vi "pylon_FSRS1.vi"() -> ()   [LabVIEW 2014]
uses:
  Public/Documents/SIToolkit/LabVIEW/Examples2014_6_0_2_9/Fast Examples/Open-Close Hardware/CamHandle.vi
  <vilib>/Utility/file.llb/Write To Spreadsheet File (I64).vi
  <vilib>/Utility/file.llb/Write To Spreadsheet File (DBL).vi
panel:
  in  "?":enum32{"CONFIGURATION", "OPERATION"}(tab)=enum."OPERATION"
  in  "Bypass Cooling":bool
  in  "Write Tab Control":T1(tab)=enum."ROI"
  in  "Frames to collect (nframe)":u32=1 min=1 step=1
  in  "Exposure":dbl min=0.0 step=0.001 format="%.3f"
  in  "Timing Mode":u32(ring)=3 items=["Free Run/Timed"=1, "External Sync"=3, "Shift per Trigger"=13]
  in  "Trigger Edge":u32(ring)=1 items=["Positive Edge"=1, "Negative Edge"=2]
  in  "Collection Mode":u32(ring)=1 items=["Focus"=1, "N-Frame"=2, "Asynchronous"=3]
  in  "Readut Mode":u16(ring)=1 items=["Full Frame"=1, "Kinetics"=10]
  in  "Temperature":dbl=-75.0 format="%.2f"
  in  "Speed":i32=-2 min=-3 step=1
  in  "Gain":i32(ring)=3 items=["Don't Change "=-1, "Low"=1, "Medium"=2, "High"=3]
  in  "Offset":i32=-1 min=-1 step=1
  in  "Readout Port":i32(ring)=2 items=["Don't Change"=-1, "Low Noise"=1, "High capacity"=2]
  in  "Open":u32
  in  "Close":u32
  in  "Shutter State":u16(ring)=3 items=["Always Closed"=1, "Open Each Exposure"=2, "Open at Begining of Acquisition"=3, "Open While Waiting for Trigger"=4]
  in  "Minium Block Size":u32=1
  in  "Number of Minimum Blocks":u32=1
  in  "Number of Clean/Clears cycles":u32
  in  "Number of Strips per Clean":u32=100
  in  "Continous Cleans":bool
  in  "Skip Serial Register Clean":bool=TRUE
  in  "Kinetics Window Height":u32
  in  "Active Y Size":u32=100
  in  "Post Y":u32=8
  in  "Pre Y":u32=8
  in  "Active X Size":u32=1340
  in  "Post X":u32
  in  "Pre X":u32
  in  "Vertical Timing Index":u32
  in  "Enable  Custom Chip":bool=TRUE
  in  "Logic Output":u16(ring)=3 items=["Not Scan / Not Reading"=1, "Shutter Open"=2, "Not Ready/Busy"=3, "Always Low"=4, "Always High"=8]
  in  "Invert":bool
  out "Y Size ROI":u32=100
  out "X Size ROI":u32=1340
  in  "Y Bin":u32=100 min=1 step=1
  in  "Y End":u32=100 min=1 step=1
  in  "Y Start":u32=1 min=1 step=1
  in  "X Bin":u32=1 min=1 step=1
  in  "X End":u32=1340 min=1 max=100000 step=1
  in  "X Start":u32=1 min=1 step=1
  in  "Error Codes":string="Ready"
  out "Frame Rate":dbl=1001.0010010010011
  out "Vertical Index":u32
  out "Custom Chip Enabled":bool
  out "Vertical Timing":dbl=3.2
  out "Readout Time":dbl=0.9989999999999999
  out "Temperature":dbl=-75.0
  out "Pixel Time":i32=500
  out "Bit Depth":i32=16
  out "ReadOut Port":i32=2
  out "ADC Offset":i32=-1
  out "ADC Gain":i32=3
  out "ADC Speed":i32=2000
  in  "error in (no error)":errorcluster
  out "error out":errorcluster
  out "Camera Handle":u32=16842752
  in  "INI Flag":bool=TRUE
  in  "Camera Number":u32=1
  in  "?":enum32{"RUN", "FOCUS", "FSRS", "SPECTROGRAPH"}(tab)=enum."FOCUS"
  in  "?":bool
  in  "Exposure Time (s)":dbl=0.004 min=0.0 step=0.001 format="%.3f"
  in  "?":bool
  in  "?":bool
  out "?":u16[](graph)
  in  "file path":path
  in  "File_name":string
  in  "# of spectrum per frame":i32
  in  "# of Frames":i32
  out "Gain":dbl=14.743310504423635
  in  "FLIP SPECTRA":bool
  in  "?":bool
  in  "?":bool
  in  "?":bool
  out "Spectra":dbl[](graph)=[0.9755300872844695, 0.9756768462539598, 0.97581696418543, 0.9762743991329165, 0.9751930768187929, 0.9752114673732061, 0.9751177936489209, 0.9764930270973735, 0.9763887386039467, 0.9749810931230943, 0.9742926745030784, 0.9759744997206772, 0.9754796564203729, 0.9761178908183206, 0.9752425241815373, 0.9766219750252831, 0.9761877743519881, 0.9761361753868542, 0.9776978491334654, 0.9779277019501946, 0.977147036323896, 0.9792513539762008, 0.9795268534910172, 0.9787884146751874, 0.9804470957694494, 0.982035881204582, 0.982528667778694, 0.9825823402901814, 0.9843882822979847, 0.9839266633595681, 0.9849468846920538, 0.9872698212511262, 0.988122544550336, 0.9877812802972845, 0.9885869980663688, 0.9900703844600179, 0.9927077538710171, 0.9932628998596844, 0.9932460798479855, 0.9935570775182174, 0.9945507204569972, 0.9951647818460134, 0.9962848374908384, 0.9972893370585736, 0.9965515155280157, 0.9984594060832435, 0.9973443014380436, 0.9989028091476645, 0.9990774165831509, 0.9983506095949803, 1.0007898394202042, 0.9991913406017616, 0.9992492731339196, 1.0010480478392645, 0.999582213532268, 0.9991496850542972, 1.0003341169724274, 1.0007777101312207, 0.9999823435413888, 1.000981058256019, 1.00207813229889, 1.0016715850846636, 1.0016509685396446, 1.0023107232087645, 1.0018617734738753, 1.002175650976147, 1.0016212316773503, 1.002062777617173, 1.002372669657128, 1.0023120696051897, 1.0022985765507009, 1.0023149704491137, 1.0021015205484045, 1.0017074421552823, 1.0023106670699446, 1.0032785517995444, 1.0018856636029874, 1.0032932634895588, 1.0028768911229609, 1.003726073257663, 1.0036399397267421, 1.0033806164078303, 1.0041437793153363, 1.0037179628801496, 1.0033493482112539, 1.0037501476114246, 1.0042959964606617, 1.0042755419219582, 1.0048754785866216, 1.0047939316440613, 1.0053694568681872, 1.0038757728966237, 1.0048674931155683, 1.0047690942831697, 1.0051252430535689, 1.0053741704915389, 1.0049524139095343, 1.0045025426639995, 1.0040228927138426, 1.0039933320314238, 1.0041510866852374, 1.0033303068586903, 1.003533250646326, 1.0027459506237124, 1.0026057826647117, 1.003260830428883, 1.0032007978706163, 1.0026495289070276, 1.0021436528670513, 1.0028330294934311, 1.00231600280275, 1.0012086967393559, 1.001014014161519, 1.0015504074851016, 1.0009696535006722, 1.0019791149958475, 1.0011346392927039, 1.0012359758891582, 0.9998570077525675, 1.0010428549273014, 1.0009149466593552, 1.0002830176584063, 0.9994048138652198, 1.0002597870365144, 1.0003278859881963, 0.9995526733478612, 0.999438177342597, 0.9998261877083351, 1.0010865765016752, 1.0000489926845766, 1.0008545626290852, 1.0008522612809412, 1.0010707079783248, 1.001090857433441, 1.0008982925251158, 1.003486669845695, 1.0047949174912858, 1.0077445761417212, 1.0120141741517803, 1.0201772595698257, 1.0322536760974164, 1.0501541199055933, 1.0754172950855931, 1.1067885797289987, 1.1374285660931862, 1.1481866653218364, 1.1326606889231363, 1.09741400039275, 1.0612674001718378, 1.0350214908693538, 1.0206930861271215, 1.0139256277018351, 1.0089963920346658, 1.0060688393052548, 1.0052123238345017, 1.0028067604394633, 1.0012638696493386, 1.0013393221695588, 0.9985981192113675, 0.9987380376267128, 0.9979073384358298, 0.9967424944898179, 0.9966884820000458, 0.9963776196534506, 0.9960720866862709, 0.9965830445533452, 0.9977931108410204, 0.9985995492168933, 0.9986199775849548, 0.9987633729071931, 0.9984312093430782, 0.9997148642087165, 0.9996065463963878, 0.9998582689274716, 1.0002110852616093, 1.0000077618826129, 1.0000489132335226, 1.0003573806378223, 0.9999187010432274, 1.001963517608326, 1.0012593397700642, 1.0018807550628366, 1.0031660227654289, 1.0020918035773498, 1.0028275747471433, 1.0028088790557186, 1.0025566510225332, 1.0023556237093005, 1.0032096086622704, 1.0017564747987622, 1.0035091544995398, 1.0017366497034703, 1.0019443199711786, 1.0020298982939733, 1.0013981641538263, 1.0010735915908218, 1.001793476880256, 1.0022368226440215, 1.0014151948414793, 1.0017759582228316, 1.0014962508125689, 1.0018072606384634, 1.0000417440167613, 1.0005621657797237, 0.9998446426790336, 0.9998454860152206, 1.0001492253861217, 0.9994421154150686, 0.9995411675602213, 0.9987441278717668, 0.9998158390779703, 0.9988418583687989, 0.9993341276421205, 0.9990993990819101, 0.9990807904190898, 0.9983948439832072, 0.9985400716676921, 0.9985927240493662, 0.9982560336788509, 0.9982625964427206, 0.9985155142344474, 0.998404835032493, 0.9979263060413635, 0.9982868928614334, 0.9973870564732009, 0.9978861496786271, 0.9978082037249373, 0.9976350693353202, 0.9978557947960519, 0.9992941525783824, 0.9975784845094273, 0.9980438675332602, 0.9973132560896502, 0.9983960703496668, 0.9975817679789122, 0.9970631933860724, 0.9968645888999441, 0.9969550208616594, 0.9968574087836076, 0.9962806908544759, 0.996370069484568, 0.9981588855574023, 0.9971286326512906, 0.9968130048156779, 0.9967659060092784, 0.9962581267842879, 0.9973137060022212, 0.9964871894740839, 0.9965162310427663, 0.996997193641602, 0.9965704833779099, 0.9963915930394757, 0.9962108827034403, 0.9960472238857022, 0.995857865398809, 0.9961579582249456, 0.9971978885120082, 0.9961331760017116, 0.996721337440865, 0.9965996253465066, 0.9965304002168622, 0.9956403635637245, 0.9955790038812106, 0.9956912830823886, 0.9949089431758003, 0.9946282645549207, 0.9934605416581226, 0.9927704057498754, 0.9935944194028669, 0.991876783433561, 0.9926946308356118, 0.9932993795948648, 0.9943894372954812, 0.9936112074994828, 0.9939246568355098, 0.9935242137901221, 0.9936503123346356, 0.9936963818576866, 0.994682882264595, 0.9937856190284484, 0.9940832926061379, 0.993164306278515, 0.9940404284685382, 0.9937880441864195, 0.9942411288661716, 0.9928753466028547, 0.9950984658310266, 0.9927277176741094, 0.9940334005450226, 0.9929660360364769, 0.9930487414589113, 0.9935365540438033, 0.9934139033392642, 0.9928950534503354, 0.9929034314029997, 0.9937174013031602, 0.9923612045121255, 0.9925908921890753, 0.9932679282052643, 0.9935763003400074, 0.9931199695791296, 0.9929887699255886, 0.9918197209507501, 0.9917853379343897, 0.9921991173870989, 0.9935339294252353, 0.9925704988068781, 0.9917055357360344, 0.992014507869348, 0.9917718012401779, 0.9909311230807839, 0.9909039735016065, 0.9896572589564085, 0.9891350823517422, 0.9894682209515745, 0.9888525713434655, 0.9909080023425957, 0.9912954671309397, 0.9935124803850233, 0.9938587756634525, 0.9946849857860757, 0.996592195888077, 0.9968503534981081, 0.9973935731820813, 0.9989584060578116, 1.0019087222262957, 1.0049043836984641, 1.0080586432045664, 1.009751294323102, 1.012303874345489, 1.0129703221236666, 1.013272938321382, 1.011503753925153, 1.0105758873330835, 1.0075438150818337, 1.0057435426202306, 1.0041342342197446, 1.0026209652997937, 1.0005848295336346, 0.9994019123146808, 0.9991868572532903, 0.9977512308696675, 0.9970075134065679, 0.9966356360857342, 0.9959060548781977, 0.9964393102123654, 0.9958649592771627, 0.9950662281056751, 0.9953116557885184, 0.9948664403448791, 0.9947278335757348, 0.9939669263212532, 0.993667523914121, 0.9945029544068963, 0.9936192521599826, 0.9921074321024335, 0.9914254678032394, 0.9903272540137805, 0.9892925938271362, 0.9887848718524774, 0.9893134788695674, 0.9882838661440005, 0.9895055869783085, 0.9891480148597968, 0.9884337022120356, 0.991156915494973, 0.9896733386520254, 0.9893394415489665, 0.9904097944203936, 0.9902381774153993, 0.9901524278073909, 0.9900581421557813, 0.9905585242206175, 0.9908406929910862, 0.9915079648120938, 0.9906566524112734, 0.9911394696363427, 0.9916113980702473, 0.9910989259973373, 0.9903792532358182, 0.9907827317977844, 0.9905977304469169, 0.991456239330327, 0.9916819598107186, 0.9914199515036257, 0.9906942610155813, 0.9926315563028391, 0.9914270997426113, 0.9915539601421401, 0.9912235268405463, 0.992088607849578, 0.9913444613666713, 0.991908492679886, 0.9915866831630165, 0.9919952301201026, 0.9932504567792872, 0.9921046559674063, 0.9924291983048888, 0.9916447610149356, 0.991848590750747, 0.9921425513517983, 0.9919714570173391, 0.9925466399620982, 0.9928838907426037, 0.9924196088955134, 0.9931616675611925, 0.9927461163593102, 0.9931309100549827, 0.9934496416081131, 0.9927927896501221, 0.9934964738267893, 0.9928551133908948, 0.9942999569046416, 0.9931792408327563, 0.9925693415358496, 0.9934360330716882, 0.9949747557474269, 0.993731157710846, 0.9938433747596407, 0.994740733427746, 0.9943609592519476, 0.9943541746199618, 0.9939486211816836, 0.992950149807933, 0.9941678883691097, 0.9943180628327398, 0.99513015651641, 0.9943919298791273, 0.9941424826530518, 0.9936525300481539, 0.9949917538640838, 0.9955375244736728, 0.9951439299329877, 0.9962050263298082, 0.9963947799134774, 0.9968244979975278, 0.9983975806265784, 1.000533927758882, 1.0029408707991847, 1.0048711521008775, 1.0068304778141166, 1.007018989034806, 1.0029759503979807, 1.0000482254275387, 0.9975549973629185, 0.9974036736573202, 0.9968789927911186, 0.9960748811206702, 0.9965189333035787, 0.995140250519678, 0.9958415984118337, 0.9949389664472165, 0.9949181303181669, 0.9952042060002814, 0.9945451790485715, 0.9952437023373856, 0.994276227548833, 0.9953156888749304, 0.9942260097126655, 0.9957965248601841, 0.9946261743510755, 0.9954561818541723, 0.9950439277931782, 0.9947499204338731, 0.9946841217392777, 0.9950829252266876, 0.9954281866903525, 0.9944531747199533, 0.9950511330771304, 0.9948849293283386, 0.9952587470138156, 0.9942422382648602, 0.9926478162749266, 0.9941745367956879, 0.9937302385520251, 0.9943405037447987, 0.9940163977879987, 0.9935998700562014, 0.9939924261400744, 0.9938600227368913, 0.9942658538803476, 0.9941555176670761, 0.9943854145798364, 0.9937595474775596, 0.9942601839347238, 0.9941192503118871, 0.9939902692064626, 0.9939594250617401, 0.9938728119504552, 0.993650669917967, 0.9946982680767041, 0.9943281028619699, 0.9939645957455999, 0.9935648856308205, 0.9941752901094008, 0.9937357059814677, 0.9933247297715599, 0.9938906929289909, 0.9941043870750722, 0.9947695896697957, 0.9926702752126659, 0.9925736732160917, 0.99412276123165, 0.993005018245409, 0.9928841805326482, 0.9928156349036281, 0.9925723613309926, 0.9918506118756122, 0.9911125441857309, 0.9907333399491967, 0.9921429405981673, 0.9905810846498307, 0.9918787814012708, 0.9920241514653586, 0.9918653459895168, 0.9915914658868445, 0.992110337597804, 0.9923605206196495, 0.992686464882264, 0.9938726051269021, 0.9934677141593928, 0.9947213941988519, 0.9939523884200137, 0.9958435480641371, 0.9960878435035664, 0.998112647651406, 0.9976058258921943, 0.9992725956143081, 1.0005451377173482, 1.002641821904002, 1.0041158281009654, 1.0073714634187072, 1.0096194442337205, 1.011401650626004, 1.013070646872337, 1.0119185527223444, 1.0099088327766466, 1.009814022494501, 1.0063825249878426, 1.0032604349198055, 1.0027766338798774, 1.000287952720255, 0.9986277641920462, 0.9980477820943987, 0.9960662676711914, 0.9967893361260675, 0.9952254802975962, 0.9939518521938141, 0.9925135524883861, 0.9926959373886529, 0.9908518984681769, 0.9911725762303055, 0.9906085031171179, 0.9904494224857862, 0.9884528287629935, 0.9887177600890857, 0.9886703754231349, 0.9881853417399994, 0.9881302842296761, 0.9880208726978792, 0.9872135553097768, 0.9871836120110088, 0.9871291081351026, 0.9865338537476699, 0.9859219777639733, 0.9869134352439242, 0.9862738473151121, 0.985608104834756, 0.9867729622891286, 0.9859698167157214, 0.984919024605055, 0.9861937432678872, 0.9848322799791898, 0.9852044388456488, 0.9853417405353183, 0.9835531029615663, 0.9844598200282393, 0.9845169921245397, 0.9843776090258691, 0.9838987127482762, 0.9826194218261648, 0.9834471979752251, 0.9829395469239401, 0.9841809517721625, 0.982740266779254, 0.9832266794850923, 0.983597461693007, 0.9839050454399203, 0.9831586562985791, 0.9832238806837683, 0.9819891319177596, 0.9830146076513276, 0.9823739806909814, 0.9834248081882394, 0.982774720138555, 0.982731503435003, 0.9825121425219699, 0.9833991472534351, 0.982186136274627, 0.9826987591820081, 0.9829784313378913, 0.9840304061865316, 0.984920420832576, 0.9848016580142605, 0.984637173220356, 0.9841012255373592, 0.9845778413710072, 0.9844496403226004, 0.9849069993604949, 0.9840818986135075, 0.9838231864024809, 0.9841145257461423, 0.9834942502404114, 0.9833176167594164, 0.9825157102760381, 0.9819735573764853, 0.9829622528276347, 0.9824945822519466, 0.9800824624551667, 0.982870582958771, 0.9825981856262659, 0.9811956732852909, 0.9822624974687129, 0.9812600672546186, 0.9811591777781735, 0.9819534555557126, 0.9806681085499535, 0.9820342971216329, 0.9813579712911087, 0.9820105505538734, 0.9812343611503167, 0.9816313053027922, 0.9820953937828902, 0.9818152492770197, 0.982330765326644, 0.9814479080657366, 0.982110291220737, 0.9806881232552964, 0.9813703402444995, 0.9821895930373158, 0.9825646178286225, 0.981722882417567, 0.9808083213760249, 0.9816826966365202, 0.9831621913409136, 0.9834519852435336, 0.9819530727831046, 0.9823086743012107, 0.9811220426873025, 0.9812482776238972, 0.9827616800346425, 0.9816851891281408, 0.9813153523769537, 0.9834752237380378, 0.9827038521339388, 0.9831869462124827, 0.9837131268255906, 0.9835637613733392, 0.9825685959375935, 0.9835166246680233, 0.9832899459313126, 0.9821619515717059, 0.9848076338921278, 0.9847424893389772, 0.9841309907479139, 0.9847567871515419, 0.9850805177341108, 0.9840332666925127, 0.9856517840958284, 0.9852222998421788, 0.9856666370667512, 0.9864656814948044, 0.9864209936998543, 0.9878172455904856, 0.9880923255936395, 0.9879512362506478, 0.9885068151698244, 0.989128852007672, 0.9887875769589333, 0.9903708567833138, 0.9900511597787641, 0.9898866071468287, 0.9910275374663167, 0.9914860580416507, 0.9925235006961411, 0.9934471447697623, 0.992608252890163, 0.9951783603126805, 0.9980690075623835, 0.9997639333483898, 1.0010665261241487, 1.002430117428686, 1.0020378147127487, 1.0024980899377627, 1.003737773795738, 1.003249051965976, 1.0002194898909202, 0.9990676595023753, 0.9997259706911115, 0.9969388880023595, 0.9957886841507878, 0.9949867408433444, 0.9953954712618904, 0.9936892062542492, 0.993787433290812, 0.9927546672218368, 0.9928893848791186, 0.9925505392102796, 0.9919471661238599, 0.9934570741748587, 0.9937581848770279, 0.9938985920841611, 0.9923185810211319, 0.9943203693140323, 0.9927044973731295, 0.9925078841695358, 0.991285249799347, 0.9925814458117747, 0.9920082293903025, 0.9921409103620292, 0.9935239939757422, 0.992042032121975, 0.991648559703939, 0.9908100594812931, 0.991996668188471, 0.992115081667455, 0.9935499502402744, 0.9921610012413922, 0.992613755742525, 0.9926860544649216, 0.9931843498730183, 0.992118950616697, 0.9931345665088376, 0.9929109347534303, 0.9930572874896546, 0.9932882948815863, 0.993410070354816, 0.9928699423061463, 0.9928931278711759, 0.9924935984745651, 0.9919420343529557, 0.9949051239072446, 0.9923959438550337, 0.9931297846797755, 0.9934610282296891, 0.9922733950845375, 0.9933423129100107, 0.993633885814162, 0.9953413726408745, 0.9956784502362345, 0.9933450393933152, 0.9939926632528363, 0.9943011106654097, 0.9936895637345653, 0.9941530739146468, 0.9936349646658799, 0.9951285340555722, 0.9950972434060573, 0.992825270720686, 0.993383955751042, 0.9945219100961133, 0.9958067541327413, 0.9956233330801973, 0.994599795734717, 0.9957142187668172, 0.9952556472687264, 0.9953656877312194, 0.9946059001794542, 0.9945539643403842, 0.9962165018925121, 0.9954940183694436, 0.9946000295948717, 0.9964193418537554, 0.9949433708136919, 0.9945754853372089, 0.9948482283130354, 0.9969224697155514, 0.9958301102585727, 0.9960699859491319, 0.994981300144576, 0.9945786563610373, 0.9951551229643493, 0.9967508501720332, 0.9963034128905163, 0.9947019215592646, 0.9965787553169893, 0.9947681378143812, 0.9981260029600254, 0.9966090075869397, 0.9966873532798938, 0.9978610764780583, 0.9969297851191489, 0.9971178057933737, 0.9976647956140443, 0.9969046818611058, 0.9971255060352899, 0.9975130234326345, 0.9960516439088403, 0.99603733180533, 0.9974251622558911, 0.9978872483995073, 0.9970739386760539, 0.99930097772978, 0.995973135092528, 0.9989070331896059, 0.9979431944896187, 0.9962574318221076, 0.998284874712051, 0.9980507065885973, 0.9985778477115815, 0.9968881257036589, 0.9979917702197649, 0.9973169278119626, 0.9974323242885285, 0.9990460618991827, 0.9967916827968758, 0.9981135977737259, 0.9978829186523762, 0.9984133201845818, 0.9973040804544807, 0.9961838114111818, 0.9975563640395146, 0.996994322790135, 0.9941276195898406, 0.9983641002927954, 0.9973307539794544, 0.9974205389337224, 0.9973560126820389, 0.9974096738250385, 0.9988189450338115, 0.9961266693760946, 0.9953281298493775, 0.9974017870532675, 0.9973856781928138, 0.9976341196873302, 0.9967046783619647, 0.9969271039427557, 0.9966967454536432, 0.9979490763684615, 0.9953698577234567, 0.9975806387238231, 0.9977016134759747, 0.9985985697493704, 0.9972305476775422, 0.9967101952847037, 0.9971668005388673, 0.9964289730529284, 0.9955644243748356, 0.9959966886630661, 0.995644758687583, 0.9961616433874917, 0.9967792446201315, 0.9955099897474771, 0.9958855279549809, 0.9954476218405081, 0.9965164632663351, 0.9950987472418618, 0.9955500463495174, 0.9960084036614891, 0.9967133506266788, 0.9949838569402805, 0.9953870910750532, 0.9957161964914851, 0.9955189418471003, 0.9952780736915173, 0.9943982047829744, 0.9958594554531327, 0.9951692159641307, 0.9972328017427001, 0.9950296264899483, 0.9953994162394338, 0.9943475666868853, 0.9952644359541133, 0.995447987953035, 0.9942957701523145, 0.994689648871326, 0.9945194145312566, 0.994398451524699, 0.9933776478611506, 0.9949624280070588, 0.9942830700740656, 0.9931776278224557, 0.9923574560898841, 0.9930554951075137, 0.9946804934635376, 0.9955965668939963, 0.9954263404790484, 0.9936251677674021, 0.9925990628645381, 0.9927432773738994, 0.9935199751181003, 0.9925849730240551, 0.9930033516252744, 0.9928205912875862, 0.9909096801217612, 0.9927703039575004, 0.9911207290263226, 0.9936811659787461, 0.9922899870293168, 0.9914100350152775, 0.9921318011951723, 0.9923914376100682, 0.9917196412768485, 0.9911298413282991, 0.9921835901118113, 0.991389162165264, 0.9900308337285773, 0.9907843437132138, 0.9907360707276159, 0.9915303321538369, 0.9910914841449963, 0.9916721085335287, 0.9905147575837829, 0.9885475299200459, 0.9889453642989275, 0.9905817815731635, 0.9902133936178602, 0.988242707738733, 0.9888230852293703, 0.9888416376753377, 0.9897403338911375, 0.9889867106471915, 0.9908277720228965, 0.9897520943960653, 0.9885535791196446, 0.9893233849009734, 0.987815837986452, 0.9878231875051255, 0.9892981374801907, 0.9873831102432441, 0.9883688597489069, 0.9870737497954729, 0.9882750727641025, 0.9892368384624726, 0.9885509311823762, 0.9877328596549173, 0.988031467066814, 0.9886629145954128, 0.9869863870033517, 0.9891492312967063, 0.9862047702357074, 0.9846632856681823, 0.9857502292131517, 0.9853621145521789, 0.9875959785273185, 0.9865328093925239, 0.9868745911941753, 0.9881208793203661, 0.9875637100247531, 0.987473573375884, 0.9846613464121071, 0.9862682448151167, 0.9859936099978158, 0.9877745806584477, 0.9872523351842334, 0.9884633919606788, 0.9878702817787882, 0.9871517835946108, 0.9873182717255755, 0.9869426138212118, 0.9870630928749186, 0.9868782191180008, 0.9866290342010844, 0.9871063632126472, 0.9870767387478339, 0.9892100304806183, 0.9856950020152947, 0.9862725203091884, 0.988963026427355, 0.98713237033965, 0.9871161785494531, 0.9887067533194143, 0.9851151639884772, 0.9872035949066793, 0.986074022015706, 0.9898358190650977, 0.9893426317428032, 0.9865967008566036, 0.9869508361679556, 0.9856394191868602, 0.9884856255992025, 0.9894815163256031, 0.9882529855875178, 0.9868192366411398, 0.9861315958941457, 0.9893630527665666, 0.9868384497720943, 0.9861536189984526, 0.9888178566241863, 0.9867579453720804, 0.987179733246874, 0.9881337364604343, 0.988627432271096, 0.9893363760375293, 0.9884977254771453, 0.9866357360169483, 0.9890432499899394, 0.9853708868622296, 0.9882718264694069, 0.9856002495340267, 0.9883093383137328, 0.9893738708532213, 0.9892222089472598, 0.9896322650924652, 0.9890899936356693, 0.9859116003714216, 0.9876200119407457, 0.9880123989427891, 0.9890238550127071, 0.9877997133543077, 0.9858156669365054, 0.988452075032815, 0.9874384552105305, 0.9852668216716264, 0.990420592763384, 0.986812319833311, 0.9872746702372613, 0.9884135283243309, 0.9898559858934276, 0.9853195046285885, 0.9882116666588994, 0.988836326416156, 0.9889951277543007, 0.9889739755936575, 0.9892999397960774, 0.9890183107271877, 0.9886904943679752, 0.9893025055256274, 0.9883530237311077, 0.9904523864862361, 0.9895924113847931, 0.9882124261702746, 0.9886951765024136, 0.9872263635916005, 0.9911316500287568, 0.9903100332934901, 0.9900921332468797, 0.9908740072799542, 0.9878369893796128, 0.9904378517826975, 0.9941283419233133, 0.9904646678151535, 0.9904861383307207, 0.9899567607865835, 0.9894396209657828, 0.9891584605747445, 0.9912651432019383, 0.9881619592777285, 0.991769579354686, 0.9897143909164129, 0.9892295794789044, 0.9919979753672009, 0.9900968712395756, 0.9903607410161109, 0.990591273311813, 0.98915183511616, 0.9909957276467207, 0.9893142228087654, 0.9914818720029506, 0.9909371177919686, 0.9899079877928816, 0.9895822415817643, 0.9902121865405016, 0.9895690295265566, 0.9875805843320437, 0.9896141479065251, 0.9904862852268639, 0.9914162763875078, 0.991266180924169, 0.9900029401520938, 0.9919999062371018, 0.9924424015884847, 0.9908311716147565, 0.9922420543168002, 0.990948525584296, 0.991385538920927, 0.9897883622343855, 0.9919614812445081, 0.9902281707455857, 0.994894236690351, 0.9909491027501054, 0.9922156201249668, 0.9902288111203057, 0.9905311413181366, 0.9938940171329753, 0.9901016036840101, 0.9915677278694006, 0.9913941890768317, 0.9909395295168169, 0.9955689263522823, 0.9922709650971144, 0.9922278347497557, 0.9909074461652106, 0.9933836875407083, 0.9939377700843446, 0.9938960186208253, 0.9915969179004076, 0.9936655476411831, 0.9919779969563804, 0.9929206399541289, 0.9921486094292173, 0.9926496485478737, 0.9912891600854369, 0.992964299640567, 0.992144221783553, 0.9939411134849978, 0.9907431243871444, 0.9936131765393752, 0.9936041064577842, 0.9937652534212517, 0.9903211389560228, 0.9917327216280427, 0.9921648683304255, 0.9951627294683641, 0.9922283830374052, 0.9943289558409931, 0.9907424411869826, 0.9955227545424469, 0.9912800745547352, 0.990673420209277, 0.9937304281797643, 0.9916714634005632, 0.9930423924184894, 0.9958545325343833, 0.9927136573955114, 0.9912896227490244, 0.9947008204846555, 0.9934107799371091, 0.9938417115243933, 0.9930422668417596, 0.9943874194176832, 0.9942539265095928, 0.99358358613357, 0.9947291666979348, 0.9907425908605572, 0.993204602660715, 0.9916709524627398, 0.9920274460533192, 0.9936766086585608, 0.9945905955117497, 0.9950847195014475, 0.9958235248305671, 0.9937034857576859, 0.9920957634794582, 0.9944005725634364, 0.9927938758452877, 0.9935960311992087, 0.9940688765091084, 0.9947011284326965, 0.9920630559207819, 0.9926178278060044, 0.9949891848842399, 0.9909971055663335, 0.9931418060555824, 0.9920755548320042, 0.9925339764023511, 0.991391464781273, 0.9954887935717076, 0.9909315027789627, 0.993356356941511, 0.994125792022422, 0.9928492382244469, 0.9924124499412162, 0.9930836474614183, 0.9957568360368506, 0.9920567116124503, 0.995949526554864, 0.9947385545568362, 0.9964578839247149, 0.9933723742979639, 0.9922669358274935, 0.9934457029333249, 0.9947183773162839, 0.9929157213426574, 0.9918681434120407, 0.9940455254836, 0.9938701377972854, 0.9951183405720802, 0.9956473514790825, 0.9934702151937861, 0.9922148914587055, 0.995510311580549, 0.9916734502187543, 0.9933575076002219, 0.9940886481726275, 0.9932584306945786, 0.9929235209872966, 0.9920596643622469, 0.993537035012101, 0.9931052323790442, 0.9932359327234979, 0.9949833835334603, 0.9951405229011836, 0.9919624443660046, 0.9976276592238483, 0.9936750289238817, 0.993409570579091, 0.9910879925312652, 0.9921357728702003, 0.9915162675385596, 0.9936030923591286, 0.9922153994045801, 0.9908575485337272, 0.9931774841303613, 0.9938872017448386, 0.994590545037957, 0.993307430337993, 0.9942723088906371, 0.991539248307689, 0.9913071886055355, 0.9939526605338713, 0.9899947024134667, 0.9963538984824989, 0.992326935160918, 0.9944721464832375, 0.9949879477759577, 0.9932585658142344, 0.9947252659633552, 0.9918392897403638, 0.9936717855188546, 0.9913585910827222, 0.9939459376987864, 0.9935785140186582, 0.9940095744502577, 0.9929867803993468, 0.9942883024814116, 0.9916508951479486, 0.9946169303410003, 0.9959076070864663, 0.9950663610916375, 0.9943206922150806, 0.9938140684907849, 0.9950494616162009, 0.993770980645202, 0.995132834379052, 0.992999131041189, 0.9930887760477737, 0.9939350396495155, 0.9917095139502041, 0.9904518285228633, 0.9910789901884679, 0.994661984192398, 0.9928873507696537, 0.9951777939207228, 0.9925060014325513, 0.9923234431420449, 0.9931051406756178, 0.9910374718917979, 0.9940782455445134, 0.9930954156738621, 0.9925965219476175, 0.9915384204239156, 0.9928793321349498, 0.9946237698843003, 0.9924329193078354, 0.9957415752854321, 0.9951194694189187, 0.9943426320897144, 0.9921634357565939, 0.9912843087353878, 0.9936166878873692, 0.9902588258846677, 0.9918777256495497, 0.9928661894424234, 0.9942934336307011, 0.9913504456199527, 0.9897445948817856, 0.9905730435130362, 0.9928026520398466, 0.9941793339815761, 0.9940404003570814, 0.9911647557778969, 0.9903376546937016, 0.9923925885780875, 0.9939915308716086, 0.9934041277202572, 0.992233211680581, 0.9930241686822162, 0.9927092973837097, 0.9914536970083173, 0.9918011794127138, 0.990454223589025, 0.9951967087809804, 0.9915125127247042, 0.9896457648823944, 0.9941661939469636, 0.9901721351134997, 0.9945975496237145, 0.9905646588912258, 0.9941808187430187, 0.9902421479159336, 0.9927895007670949, 0.9912021052028566, 0.9940501892508105, 0.9910699795786526, 0.9902489427350967, 0.9923014835244222, 0.9939603840687568, 0.9954110009966485, 0.9910917139952687, 0.9900019962556841, 0.9911081561325191, 0.9923107852154391, 0.9912133177459406, 0.9904204625520502, 0.9936610095017795, 0.9896768258723022, 0.9923443297455112, 0.9917565335671285, 0.9905687625686151, 0.9888984774901507, 0.9893084530792791, 0.9933156396520979, 0.9919936194580224, 0.9890713034236597, 0.9926432419634252, 0.9905729663389071, 0.9902960594148464, 0.9876980881417844, 0.9919849025918183, 0.9906527359482012, 0.9906389184677282, 0.9898359762578668, 0.992066980288709, 0.9881393391249601, 0.9882547917192857, 0.9886340003533658, 0.9909012595462037, 0.9893503136176642, 0.9876874518723383, 0.9901566948143121, 0.9908113988992338, 0.991077329668877, 0.9913905420699904, 0.9910538349777066, 0.9904577062540806, 0.9901097601524909, 0.9888310537365281]
  in  "?":bool
  out "?":dbl[](graph)=[11117.479591836734, 11148.581632653062, 11117.285714285714, 11113.479591836734, 11133.489795918367, 11164.632653061224, 11197.051020408164, 11198.489795918367, 11219.540816326531, 11280.989795918367, 11300.969387755102, 11356.397959183674, 11402.785714285714, 11438.336734693878, 11505.34693877551, 11556.632653061224, 11603.183673469388, 11680.214285714286, 11759.438775510203, 11832.418367346938, 11956.07142857143, 12034.081632653062, 12139.5, 12209.19387755102, 12348.408163265307, 12462.948979591836, 12583.877551020409, 12736.5, 12793.908163265307, 12993.591836734693, 13161.948979591836, 13306.765306122448, 13460.387755102041, 13578.214285714286, 13758.561224489797, 13935.285714285714, 14158.34693877551, 14246.408163265307, 14480.69387755102, 14598.357142857143, 14785.591836734693, 14938.214285714286, 15152.918367346938, 15356.214285714286, 15482.989795918367, 15698.765306122448, 15814.979591836734, 16026.030612244898, 16304.938775510203, 16417.785714285714, 16571.214285714286, 16764.928571428572, 16962.79591836735, 17180.30612244898, 17237.15306122449, 17463.061224489797, 17692.877551020407, 17915.877551020407, 18028.285714285714, 18207.367346938776, 18485.14285714286, 18716.65306122449, 18942.071428571428, 19127.65306122449, 19350.867346938776, 19535.908163265307, 19644.224489795917, 19865.214285714286, 19952.918367346938, 20267.64285714286, 20405.744897959183, 20655.908163265307, 20863.23469387755, 21031.336734693876, 21199.397959183672, 21422.79591836735, 21701.816326530614, 21831.520408163266, 22000.602040816328, 22165.816326530614, 22370.80612244898, 22493.23469387755, 22693.581632653062, 22827.571428571428, 22933.408163265307, 23189.030612244896, 23285.469387755104, 23409.29591836735, 23638.84693877551, 23869.15306122449, 23950.173469387755, 24075.38775510204, 24271.45918367347, 24375.173469387755, 24540.316326530614, 24618.020408163266, 24800.183673469386, 24912.591836734693, 24900.928571428572, 24985.724489795917, 25119.571428571428, 25268.673469387755, 25418.448979591838, 25529.45918367347, 25554.714285714286, 25682.397959183672, 25724.122448979593, 25839.020408163266, 25923.918367346938, 26014.479591836734, 25964.744897959183, 26110.64285714286, 26152.724489795917, 26314.469387755104, 26328.26530612245, 26517.14285714286, 26494.785714285714, 26658.285714285714, 26614.69387755102, 26718.80612244898, 26744.367346938776, 26752.26530612245, 26833.26530612245, 26912.755102040817, 26918.14285714286, 26999.755102040817, 27018.214285714286, 27066.377551020407, 27104.061224489797, 27109.173469387755, 27222.744897959183, 27361.34693877551, 27252.571428571428, 27353.969387755104, 27311.775510204083, 27497.918367346938, 27534.224489795917, 27719.34693877551, 27903.214285714286, 28103.826530612245, 28533.755102040817, 28986.081632653062, 29831.285714285714, 30749.602040816328, 31593.163265306124, 31919.836734693876, 31631.683673469386, 30499.622448979593, 29614.030612244896, 28945.785714285714, 28654.20408163265, 28425.428571428572, 28381.79591836735, 28224.602040816328, 28374.64285714286, 28273.530612244896, 28239.591836734693, 28174.224489795917, 28258.928571428572, 28291.244897959183, 28264.061224489797, 28282.897959183672, 28273.081632653062, 28443.326530612245, 28421.20408163265, 28422.408163265307, 28489.326530612245, 28506.51020408163, 28532.397959183672, 28600.408163265307, 28633.632653061224, 28850.908163265307, 28747.61224489796, 28736.377551020407, 28547.20408163265, 28556.724489795917, 28256.69387755102, 28239.775510204083, 28131.15306122449, 28556.418367346938, 28786.724489795917, 29128.84693877551, 29035.479591836734, 28962.98979591837, 29099.938775510203, 28978.071428571428, 29061.438775510203, 29083.836734693876, 28999.581632653062, 29001.928571428572, 28930.071428571428, 28918.88775510204, 28895.285714285714, 28825.15306122449, 28937.979591836734, 28762.326530612245, 28719.73469387755, 28861.255102040817, 28881.122448979593, 28736.183673469386, 28760.14285714286, 28713.183673469386, 28589.45918367347, 28575.836734693876, 28519.397959183672, 28374.54081632653, 28524.785714285714, 28372.030612244896, 28348.561224489797, 28258.377551020407, 28274.35714285714, 28046.54081632653, 28039.84693877551, 28163.51020408163, 27994.418367346938, 27789.84693877551, 27786.724489795917, 27765.316326530614, 27687.19387755102, 27616.275510204083, 27594.632653061224, 27495.30612244898, 27333.602040816328, 27321.918367346938, 27214.5, 27084.84693877551, 27027.663265306124, 26885.01020408163, 26820.724489795917, 26843.80612244898, 26775.897959183672, 26582.755102040817, 26468.01020408163, 26509.448979591838, 26347.38775510204, 26246.70408163265, 26076.19387755102, 25936.020408163266, 25814.45918367347, 25805.5, 25693.73469387755, 25635.724489795917, 25643.23469387755, 25456.20408163265, 25285.0, 25352.867346938776, 25215.285714285714, 25146.591836734693, 25130.948979591838, 24985.98979591837, 24843.122448979593, 24791.102040816328, 24754.530612244896, 24654.520408163266, 24542.73469387755, 24495.04081632653, 24487.877551020407, 24404.979591836734, 24295.23469387755, 24306.714285714286, 24226.5, 24179.785714285714, 24306.724489795917, 24099.04081632653, 23980.316326530614, 23929.95918367347, 23730.377551020407, 23668.867346938776, 23663.04081632653, 23568.80612244898, 23642.928571428572, 23677.14285714286, 23708.030612244896, 23678.214285714286, 23698.755102040817, 23720.5, 23686.683673469386, 23594.79591836735, 23615.724489795917, 23637.581632653062, 23593.775510204083, 23561.724489795917, 23602.79591836735, 23572.61224489796, 23665.64285714286, 23609.5, 23745.73469387755, 23638.469387755104, 23652.622448979593, 23733.377551020407, 23601.816326530614, 23709.95918367347, 23671.938775510203, 23769.255102040817, 23770.23469387755, 23820.448979591838, 23872.714285714286, 23844.561224489797, 23855.663265306124, 23952.173469387755, 24046.571428571428, 24066.367346938776, 24019.79591836735, 24093.571428571428, 24201.469387755104, 24149.64285714286, 24295.95918367347, 24328.061224489797, 24342.15306122449, 24263.551020408162, 24326.561224489797, 24392.336734693876, 24424.867346938776, 24423.285714285714, 24604.20408163265, 24561.34693877551, 24681.418367346938, 24709.530612244896, 24809.714285714286, 24964.95918367347, 24936.84693877551, 25144.0, 25134.581632653062, 25251.938775510203, 25463.418367346938, 25449.51020408163, 25539.30612244898, 25647.979591836734, 25671.918367346938, 25948.15306122449, 25938.316326530614, 26008.01020408163, 25879.744897959183, 25930.867346938776, 25914.0, 25994.908163265307, 25986.61224489796, 25921.908163265307, 25880.38775510204, 25863.673469387755, 25875.29591836735, 25818.632653061224, 25923.54081632653, 25936.091836734693, 25999.244897959183, 26021.071428571428, 26009.14285714286, 25969.214285714286, 25993.01020408163, 26054.897959183672, 26051.479591836734, 26117.714285714286, 26112.663265306124, 26145.11224489796, 26081.530612244896, 26133.316326530614, 25987.34693877551, 25937.54081632653, 25816.01020408163, 25827.755102040817, 25816.622448979593, 25921.061224489797, 25936.775510204083, 25893.367346938776, 25838.64285714286, 25916.673469387755, 25835.755102040817, 25762.79591836735, 25805.908163265307, 25872.938775510203, 25784.95918367347, 25777.377551020407, 25778.030612244896, 25684.418367346938, 25657.45918367347, 25643.80612244898, 25724.663265306124, 25678.581632653062, 25573.35714285714, 25522.48979591837, 25438.132653061224, 25530.30612244898, 25451.622448979593, 25501.183673469386, 25403.591836734693, 25445.34693877551, 25249.428571428572, 25292.020408163266, 25163.275510204083, 25219.448979591838, 25228.928571428572, 25187.26530612245, 25009.51020408163, 25012.867346938776, 24963.367346938776, 24965.132653061224, 25032.244897959183, 24837.29591836735, 24733.826530612245, 24726.35714285714, 24605.51020408163, 24638.438775510203, 24518.448979591838, 24446.34693877551, 24473.244897959183, 24386.683673469386, 24281.551020408162, 24220.214285714286, 24227.673469387755, 24137.408163265307, 24145.61224489796, 24068.98979591837, 24080.65306122449, 23838.0, 23783.20408163265, 23869.30612244898, 23785.877551020407, 23709.836734693876, 23704.673469387755, 23696.30612244898, 23523.45918367347, 23475.561224489797, 23415.54081632653, 23327.051020408162, 23326.397959183672, 23354.26530612245, 23138.081632653062, 23120.020408163266, 23100.775510204083, 22950.173469387755, 22903.571428571428, 22895.15306122449, 22820.04081632653, 22736.51020408163, 22625.29591836735, 22687.5, 22597.979591836734, 22531.326530612245, 22484.561224489797, 22550.19387755102, 22479.224489795917, 22433.255102040817, 22269.775510204083, 22051.98979591837, 21983.897959183672, 21933.183673469386, 21822.520408163266, 21831.316326530614, 21735.030612244896, 21653.755102040817, 21636.683673469386, 21628.918367346938, 21479.64285714286, 21433.081632653062, 21354.26530612245, 21255.23469387755, 21177.102040816328, 21186.80612244898, 21072.285714285714, 21047.479591836734, 20957.520408163266, 20912.755102040817, 20813.214285714286, 20794.70408163265, 20741.35714285714, 20707.26530612245, 20568.65306122449, 20525.744897959183, 20503.0, 20382.479591836734, 20364.122448979593, 20319.336734693876, 20191.448979591838, 20167.84693877551, 20086.785714285714, 20004.173469387755, 19987.20408163265, 19951.01020408163, 19873.591836734693, 19792.979591836734, 19710.469387755104, 19658.64285714286, 19473.163265306124, 19428.88775510204, 19436.316326530614, 19363.061224489797, 19302.571428571428, 19223.775510204083, 19127.051020408162, 19197.326530612245, 19028.51020408163, 18937.867346938776, 18845.591836734693, 18811.071428571428, 18781.38775510204, 18711.724489795917, 18624.95918367347, 18586.408163265307, 18514.173469387755, 18425.88775510204, 18399.561224489797, 18284.479591836734, 18320.061224489797, 18168.836734693876, 17972.602040816328, 17731.520408163266, 17431.428571428572, 17301.183673469386, 17272.714285714286, 17389.224489795917, 17490.336734693876, 17494.5, 17450.01020408163, 17346.867346938776, 17267.244897959183, 17232.70408163265, 17217.73469387755, 17155.15306122449, 17025.15306122449, 17027.020408163266, 16975.785714285714, 16863.744897959183, 16800.336734693876, 16747.285714285714, 16664.64285714286, 16597.102040816328, 16563.30612244898, 16453.908163265307, 16402.122448979593, 16401.081632653062, 16345.112244897959, 16387.183673469386, 16329.438775510203, 16292.42857142857, 16239.673469387755, 16209.836734693878, 16069.224489795919, 16011.275510204081, 15872.724489795919, 15785.091836734693, 15717.234693877552, 15582.5, 15502.867346938776, 15468.918367346938, 15348.92857142857, 15274.581632653062, 15246.591836734693, 15130.591836734693, 15074.540816326531, 14953.602040816326, 14924.948979591836, 14894.15306122449, 14811.816326530612, 14722.5, 14727.183673469388, 14656.908163265307, 14593.591836734693, 14497.336734693878, 14463.19387755102, 14433.275510204081, 14363.0, 14278.816326530612, 14261.020408163266, 14230.367346938776, 14170.989795918367, 14153.336734693878, 14015.132653061224, 14029.744897959185, 13932.581632653062, 13879.102040816326, 13829.887755102041, 13797.540816326531, 13740.387755102041, 13710.663265306122, 13666.336734693878, 13618.357142857143, 13557.367346938776, 13478.326530612245, 13452.510204081633, 13427.275510204081, 13424.387755102041, 13327.061224489797, 13296.397959183674, 13308.183673469388, 13293.336734693878, 13226.224489795919, 13213.581632653062, 13169.57142857143, 13060.765306122448, 13040.387755102041, 13015.5, 12955.69387755102, 12938.112244897959, 12937.15306122449, 12887.918367346938, 12826.448979591836, 12813.877551020409, 12781.30612244898, 12801.69387755102, 12729.673469387755, 12639.724489795919, 12662.459183673469, 12632.591836734693, 12633.42857142857, 12588.459183673469, 12624.612244897959, 12562.010204081633, 12524.704081632653, 12466.969387755102, 12383.836734693878, 12391.591836734693, 12381.867346938776, 12383.265306122448, 12358.326530612245, 12364.275510204081, 12290.84693877551, 12254.602040816326, 12200.69387755102, 12194.30612244898, 12188.5, 12168.234693877552, 12182.887755102041, 12126.765306122448, 12105.683673469388, 12112.948979591836, 12063.948979591836, 12010.785714285714, 12025.295918367347, 11991.5, 12024.69387755102, 11940.295918367347, 11903.19387755102, 11917.540816326531, 11923.30612244898, 11877.948979591836, 11857.80612244898, 11838.459183673469, 11800.255102040815, 11832.0, 11780.418367346938, 11755.908163265307, 11712.816326530612, 11705.642857142857, 11699.92857142857, 11687.897959183674, 11653.408163265307, 11554.040816326531, 11560.612244897959, 11525.42857142857, 11556.897959183674, 11511.581632653062, 11504.34693877551, 11445.561224489797, 11480.65306122449, 11457.142857142857, 11422.265306122448, 11420.510204081633, 11347.081632653062, 11330.755102040815, 11358.908163265307, 11302.367346938776, 11268.57142857143, 11300.92857142857, 11242.15306122449, 11228.418367346938, 11199.908163265307, 11161.0, 11101.30612244898, 11092.061224489797, 11149.673469387755, 11098.15306122449, 11049.989795918367, 10989.367346938776, 11016.897959183674, 11033.091836734693, 10986.795918367347, 10984.540816326531, 10968.469387755102, 10920.408163265307, 10899.959183673469, 10872.336734693878, 10852.520408163266, 10841.367346938776, 10842.122448979591, 10812.989795918367, 10820.377551020409, 10745.448979591836, 10764.540816326531, 10771.80612244898, 10739.897959183674, 10662.204081632653, 10631.683673469388, 10577.469387755102, 10536.19387755102, 10555.244897959185, 10502.316326530612, 10503.673469387755, 10455.918367346938, 10453.285714285714, 10377.581632653062, 10397.673469387755, 10379.397959183674, 10360.826530612245, 10348.214285714286, 10320.418367346938, 10262.959183673469, 10188.673469387755, 10159.959183673469, 10168.081632653062, 10127.19387755102, 10121.234693877552, 10098.112244897959, 10077.061224489797, 10012.19387755102, 9963.826530612245, 9940.714285714286, 9943.387755102041, 9920.040816326531, 9849.65306122449, 9868.275510204081, 9814.591836734693, 9703.0, 9706.714285714286, 9695.683673469388, 9688.122448979591, 9669.489795918367, 9653.765306122448, 9595.408163265307, 9549.622448979591, 9503.397959183674, 9485.061224489797, 9454.418367346938, 9457.0, 9409.510204081633, 9360.42857142857, 9343.969387755102, 9326.632653061224, 9283.867346938776, 9258.377551020409, 9198.19387755102, 9125.265306122448, 9138.663265306122, 9144.19387755102, 9133.112244897959, 9094.724489795919, 9043.948979591836, 9035.010204081633, 9001.581632653062, 8979.42857142857, 8948.602040816326, 8948.5, 8903.632653061224, 8852.632653061224, 8775.948979591836, 8780.418367346938, 8731.663265306122, 8706.959183673469, 8688.0, 8618.979591836734, 8616.438775510203, 8572.520408163266, 8545.42857142857, 8498.65306122449, 8473.867346938776, 8464.948979591836, 8445.84693877551, 8388.989795918367, 8353.959183673469, 8337.918367346938, 8311.183673469388, 8265.591836734693, 8240.19387755102, 8194.642857142857, 8201.561224489797, 8164.4795918367345, 8124.714285714285, 8100.7040816326535, 8049.836734693878, 8033.734693877551, 7995.622448979592, 7961.071428571428, 7911.857142857143, 7903.2040816326535, 7852.0204081632655, 7834.785714285715, 7815.0, 7769.622448979592, 7781.15306122449, 7730.683673469388, 7668.765306122449, 7643.0204081632655, 7642.867346938776, 7616.5, 7559.336734693878, 7548.265306122449, 7519.030612244898, 7489.571428571428, 7442.173469387755, 7407.877551020408, 7381.010204081633, 7349.765306122449, 7319.265306122449, 7305.826530612245, 7282.306122448979, 7239.122448979592, 7195.632653061224, 7158.908163265306, 7172.285714285715, 7143.102040816327, 7126.336734693878, 7100.316326530612, 7040.102040816327, 7015.622448979592, 6994.367346938776, 6970.928571428572, 6929.867346938776, 6889.122448979592, 6835.918367346939, 6853.326530612245, 6810.193877551021, 6765.091836734694, 6767.367346938776, 6719.744897959184, 6682.438775510204, 6688.561224489796, 6642.0, 6631.928571428572, 6605.5, 6593.102040816327, 6578.683673469388, 6542.469387755102, 6497.408163265306, 6490.4795918367345, 6457.1122448979595, 6426.908163265306, 6400.530612244898, 6351.724489795918, 6340.244897959184, 6314.551020408163, 6296.122448979592, 6283.755102040816, 6266.418367346939, 6239.367346938776, 6211.734693877551, 6168.336734693878, 6162.775510204082, 6132.724489795918, 6104.173469387755, 6089.928571428572, 6037.622448979592, 6023.9795918367345, 5993.714285714285, 5974.244897959184, 5947.7040816326535, 5921.714285714285, 5906.051020408163, 5865.244897959184, 5861.877551020408, 5821.030612244898, 5809.65306122449, 5799.316326530612, 5778.714285714285, 5739.2040816326535, 5724.989795918367, 5695.4795918367345, 5676.724489795918, 5655.84693877551, 5642.816326530612, 5634.285714285715, 5593.581632653061, 5578.551020408163, 5555.010204081633, 5545.693877551021, 5536.806122448979, 5499.3877551020405, 5467.367346938776, 5442.081632653061, 5435.683673469388, 5399.561224489796, 5396.510204081633, 5377.1122448979595, 5357.408163265306, 5327.642857142857, 5312.316326530612, 5311.244897959184, 5276.867346938776, 5257.5204081632655, 5249.326530612245, 5226.214285714285, 5185.959183673469, 5163.959183673469, 5155.040816326531, 5138.255102040816, 5121.938775510204, 5101.193877551021, 5095.163265306122, 5059.551020408163, 5045.469387755102, 5026.15306122449, 5013.5204081632655, 5011.724489795918, 5001.030612244898, 4957.255102040816, 4931.602040816327, 4945.0204081632655, 4926.581632653061, 4912.163265306122, 4889.744897959184, 4874.7959183673465, 4857.183673469388, 4844.234693877551, 4827.102040816327, 4809.071428571428, 4789.9795918367345, 4774.744897959184, 4750.836734693878, 4745.285714285715, 4729.224489795918, 4717.673469387755, 4686.091836734694, 4685.489795918367, 4658.571428571428, 4640.989795918367, 4643.459183673469, 4613.826530612245, 4595.459183673469, 4574.357142857143, 4563.571428571428, 4555.551020408163, 4514.897959183673, 4495.714285714285, 4446.34693877551, 4468.642857142857, 4483.948979591837, 4469.6122448979595, 4446.2959183673465, 4429.744897959184, 4388.826530612245, 4327.1122448979595, 4276.255102040816, 4338.489795918367, 4336.265306122449, 4329.234693877551, 4321.7959183673465, 4313.561224489796, 4281.234693877551, 4253.173469387755, 4224.581632653061, 4169.724489795918, 4176.438775510204, 4192.897959183673, 4168.091836734694, 4176.673469387755, 4166.897959183673, 4162.84693877551, 4132.642857142857, 4108.336734693878, 4059.173469387755, 4016.8979591836733, 4053.030612244898, 4057.9489795918366, 4034.591836734694, 4029.908163265306, 3993.3469387755104, 3947.8979591836733, 3988.734693877551, 3931.0408163265306, 3859.8673469387754, 3819.581632653061, 3820.9285714285716, 3842.326530612245, 3818.8061224489797, 3890.9591836734694, 3899.326530612245, 3875.4795918367345, 3892.7755102040815, 3870.234693877551, 3854.816326530612, 3823.8367346938776, 3771.234693877551, 3700.622448979592, 3733.1632653061224, 3772.265306122449, 3746.061224489796, 3675.714285714286, 3687.5714285714284, 3732.0408163265306, 3727.1428571428573, 3736.326530612245, 3703.908163265306, 3699.8061224489797, 3686.173469387755, 3649.377551020408, 3632.1530612244896, 3621.9795918367345, 3629.061224489796, 3623.2244897959185, 3572.5714285714284, 3573.765306122449, 3502.214285714286, 3512.9285714285716, 3573.2551020408164, 3551.581632653061, 3547.6020408163267, 3540.1632653061224, 3507.5510204081634, 3444.1938775510203, 3467.408163265306, 3480.4591836734694, 3460.173469387755, 3388.795918367347, 3432.183673469388, 3445.3367346938776, 3426.8061224489797, 3437.3979591836733, 3412.5714285714284, 3372.6326530612246, 3370.5714285714284, 3398.6326530612246, 3375.6632653061224, 3379.612244897959, 3363.918367346939, 3351.2551020408164, 3326.3673469387754, 3321.438775510204, 3311.2551020408164, 3302.5714285714284, 3295.1938775510203, 3271.8061224489797, 3254.908163265306, 3231.122448979592, 3221.561224489796, 3223.4285714285716, 3214.0204081632655, 3201.5510204081634, 3187.6938775510203, 3177.326530612245, 3171.734693877551, 3163.6428571428573, 3145.5, 3152.4795918367345, 3126.7244897959185, 3098.9591836734694, 3083.5510204081634, 3093.1530612244896, 3074.826530612245, 3071.714285714286, 3051.785714285714, 3050.234693877551, 3015.204081632653, 2987.3673469387754, 2996.816326530612, 3000.7551020408164, 2982.3571428571427, 2967.091836734694, 2935.622448979592, 2938.173469387755, 2932.938775510204, 2921.9795918367345, 2896.469387755102, 2837.795918367347, 2794.9897959183672, 2781.1530612244896, 2817.826530612245, 2830.7551020408164, 2808.8061224489797, 2823.0408163265306, 2823.0204081632655, 2813.4795918367345, 2790.8061224489797, 2786.1530612244896, 2777.969387755102, 2736.785714285714, 2712.7755102040815, 2725.877551020408, 2686.908163265306, 2601.1020408163267, 2655.4591836734694, 2678.5, 2662.9795918367345, 2661.826530612245, 2655.6326530612246, 2647.295918367347, 2644.7448979591836, 2643.2448979591836, 2632.204081632653, 2614.2448979591836, 2604.6632653061224, 2596.0408163265306, 2591.887755102041, 2567.918367346939, 2545.785714285714, 2528.0510204081634, 2507.8061224489797, 2530.877551020408, 2527.1530612244896, 2500.316326530612, 2478.1938775510203, 2449.969387755102, 2464.214285714286, 2469.7448979591836, 2467.214285714286, 2455.0, 2447.8367346938776, 2443.6020408163267, 2425.2448979591836, 2412.6020408163267, 2407.081632653061, 2382.8979591836733, 2395.887755102041, 2395.3061224489797, 2379.8061224489797, 2366.091836734694, 2360.5510204081634, 2344.387755102041, 2337.3979591836733, 2340.7551020408164, 2337.673469387755, 2313.204081632653, 2298.030612244898, 2267.4489795918366, 2234.183673469388, 2246.1020408163267, 2276.734693877551, 2277.765306122449, 2256.2244897959185, 2247.4285714285716, 2239.918367346939, 2235.714285714286, 2231.316326530612, 2219.377551020408, 2211.938775510204, 2205.091836734694, 2186.265306122449, 2178.4591836734694, 2135.091836734694, 2142.8673469387754, 2151.9591836734694, 2146.091836734694, 2137.112244897959, 2131.173469387755, 2124.091836734694, 2099.2755102040815, 2071.295918367347, 2093.683673469388, 2094.1632653061224, 2098.3673469387754, 2095.918367346939, 2084.673469387755, 2083.2244897959185, 2068.8061224489797, 2066.1020408163267, 2059.3979591836733, 2051.8979591836733, 2044.8163265306123, 2035.2142857142858, 2025.9285714285713, 2028.5408163265306, 2014.7448979591836, 2007.1020408163265, 1981.857142857143, 1975.0714285714287, 1981.3469387755101, 1972.6224489795918, 1975.295918367347, 1963.2448979591836, 1943.3367346938776, 1938.408163265306, 1953.9285714285713, 1942.6632653061224, 1932.6530612244899, 1937.5510204081634, 1927.2857142857142, 1920.295918367347, 1911.1530612244899, 1914.1122448979593, 1912.2857142857142, 1908.3367346938776, 1901.1326530612246, 1888.469387755102, 1885.1836734693877, 1876.7755102040817, 1865.2142857142858, 1868.2448979591836, 1861.969387755102, 1855.8367346938776, 1853.6734693877552, 1845.5714285714287, 1837.3979591836735, 1823.5102040816328, 1805.9795918367347, 1799.4897959183672, 1813.8469387755101, 1808.857142857143, 1807.938775510204, 1802.2755102040817, 1790.642857142857, 1787.9591836734694, 1782.3673469387754, 1776.0408163265306, 1772.4285714285713, 1747.9897959183672, 1747.5102040816328, 1743.0714285714287, 1743.4285714285713, 1739.3265306122448, 1727.530612244898, 1727.5510204081634, 1721.4183673469388, 1719.3673469387754, 1711.1020408163265, 1698.969387755102, 1697.357142857143, 1683.142857142857, 1681.3979591836735, 1671.8265306122448, 1660.8061224489795, 1665.1224489795918, 1660.1326530612246, 1658.734693877551, 1649.7551020408164, 1643.8979591836735, 1638.3061224489795, 1635.1122448979593, 1634.908163265306, 1623.765306122449, 1619.765306122449, 1617.642857142857, 1613.1938775510205, 1601.8061224489795, 1587.5714285714287, 1578.5, 1579.9285714285713, 1579.2857142857142, 1571.734693877551, 1563.8979591836735, 1560.0, 1558.1122448979593, 1547.561224489796, 1540.5408163265306, 1532.8979591836735, 1530.3163265306123, 1525.8673469387754, 1523.7448979591836, 1515.857142857143, 1512.704081632653, 1508.7755102040817, 1506.4183673469388, 1503.3367346938776, 1496.5, 1489.8469387755101, 1488.530612244898, 1482.5102040816328, 1475.5510204081634, 1473.5510204081634, 1472.5204081632653, 1468.204081632653, 1453.9897959183672, 1447.4285714285713, 1445.469387755102, 1443.9183673469388, 1433.5408163265306, 1434.4591836734694, 1430.4591836734694, 1426.7857142857142, 1416.3673469387754, 1415.704081632653, 1409.6326530612246, 1409.561224489796, 1402.908163265306, 1394.3163265306123, 1389.357142857143, 1387.7857142857142, 1390.6326530612246, 1382.3061224489795, 1369.1632653061224, 1366.3265306122448, 1366.4285714285713, 1364.969387755102, 1351.2448979591836, 1353.0408163265306, 1350.7551020408164, 1348.438775510204, 1343.9795918367347, 1337.295918367347, 1337.765306122449, 1331.3469387755101, 1330.3265306122448, 1315.9795918367347, 1319.0102040816328, 1314.265306122449, 1311.6530612244899, 1303.2857142857142, 1299.234693877551, 1292.8265306122448, 1289.938775510204, 1289.357142857143, 1281.1326530612246, 1282.2448979591836, 1280.969387755102, 1271.9897959183672, 1266.3979591836735, 1269.9285714285713, 1259.5816326530612, 1259.4285714285713, 1258.3979591836735, 1252.0408163265306, 1247.9591836734694, 1247.8265306122448, 1240.469387755102, 1231.8061224489795, 1233.0714285714287, 1231.1734693877552, 1228.908163265306, 1222.8061224489795, 1222.2244897959183, 1215.591836734694, 1213.295918367347, 1207.9795918367347, 1201.0714285714287, 1203.9795918367347, 1201.8877551020407, 1193.6632653061224, 1192.4489795918366, 1189.5816326530612, 1185.9591836734694, 1182.0, 1177.8469387755101, 1170.061224489796, 1166.765306122449, 1173.091836734694, 1160.2142857142858, 1157.1224489795918, 1160.5714285714287, 1154.8877551020407, 1146.795918367347, 1143.0102040816328, 1139.561224489796]
  out "?":dbl[](graph)=[11117.479591836734, 11148.581632653062, 11117.285714285714, 11113.479591836734, 11133.489795918367, 11164.632653061224, 11197.051020408164, 11198.489795918367, 11219.540816326531, 11280.989795918367, 11300.969387755102, 11356.397959183674, 11402.785714285714, 11438.336734693878, 11505.34693877551, 11556.632653061224, 11603.183673469388, 11680.214285714286, 11759.438775510203, 11832.418367346938, 11956.07142857143, 12034.081632653062, 12139.5, 12209.19387755102, 12348.408163265307, 12462.948979591836, 12583.877551020409, 12736.5, 12793.908163265307, 12993.591836734693, 13161.948979591836, 13306.765306122448, 13460.387755102041, 13578.214285714286, 13758.561224489797, 13935.285714285714, 14158.34693877551, 14246.408163265307, 14480.69387755102, 14598.357142857143, 14785.591836734693, 14938.214285714286, 15152.918367346938, 15356.214285714286, 15482.989795918367, 15698.765306122448, 15814.979591836734, 16026.030612244898, 16304.938775510203, 16417.785714285714, 16571.214285714286, 16764.928571428572, 16962.79591836735, 17180.30612244898, 17237.15306122449, 17463.061224489797, 17692.877551020407, 17915.877551020407, 18028.285714285714, 18207.367346938776, 18485.14285714286, 18716.65306122449, 18942.071428571428, 19127.65306122449, 19350.867346938776, 19535.908163265307, 19644.224489795917, 19865.214285714286, 19952.918367346938, 20267.64285714286, 20405.744897959183, 20655.908163265307, 20863.23469387755, 21031.336734693876, 21199.397959183672, 21422.79591836735, 21701.816326530614, 21831.520408163266, 22000.602040816328, 22165.816326530614, 22370.80612244898, 22493.23469387755, 22693.581632653062, 22827.571428571428, 22933.408163265307, 23189.030612244896, 23285.469387755104, 23409.29591836735, 23638.84693877551, 23869.15306122449, 23950.173469387755, 24075.38775510204, 24271.45918367347, 24375.173469387755, 24540.316326530614, 24618.020408163266, 24800.183673469386, 24912.591836734693, 24900.928571428572, 24985.724489795917, 25119.571428571428, 25268.673469387755, 25418.448979591838, 25529.45918367347, 25554.714285714286, 25682.397959183672, 25724.122448979593, 25839.020408163266, 25923.918367346938, 26014.479591836734, 25964.744897959183, 26110.64285714286, 26152.724489795917, 26314.469387755104, 26328.26530612245, 26517.14285714286, 26494.785714285714, 26658.285714285714, 26614.69387755102, 26718.80612244898, 26744.367346938776, 26752.26530612245, 26833.26530612245, 26912.755102040817, 26918.14285714286, 26999.755102040817, 27018.214285714286, 27066.377551020407, 27104.061224489797, 27109.173469387755, 27222.744897959183, 27361.34693877551, 27252.571428571428, 27353.969387755104, 27311.775510204083, 27497.918367346938, 27534.224489795917, 27719.34693877551, 27903.214285714286, 28103.826530612245, 28533.755102040817, 28986.081632653062, 29831.285714285714, 30749.602040816328, 31593.163265306124, 31919.836734693876, 31631.683673469386, 30499.622448979593, 29614.030612244896, 28945.785714285714, 28654.20408163265, 28425.428571428572, 28381.79591836735, 28224.602040816328, 28374.64285714286, 28273.530612244896, 28239.591836734693, 28174.224489795917, 28258.928571428572, 28291.244897959183, 28264.061224489797, 28282.897959183672, 28273.081632653062, 28443.326530612245, 28421.20408163265, 28422.408163265307, 28489.326530612245, 28506.51020408163, 28532.397959183672, 28600.408163265307, 28633.632653061224, 28850.908163265307, 28747.61224489796, 28736.377551020407, 28547.20408163265, 28556.724489795917, 28256.69387755102, 28239.775510204083, 28131.15306122449, 28556.418367346938, 28786.724489795917, 29128.84693877551, 29035.479591836734, 28962.98979591837, 29099.938775510203, 28978.071428571428, 29061.438775510203, 29083.836734693876, 28999.581632653062, 29001.928571428572, 28930.071428571428, 28918.88775510204, 28895.285714285714, 28825.15306122449, 28937.979591836734, 28762.326530612245, 28719.73469387755, 28861.255102040817, 28881.122448979593, 28736.183673469386, 28760.14285714286, 28713.183673469386, 28589.45918367347, 28575.836734693876, 28519.397959183672, 28374.54081632653, 28524.785714285714, 28372.030612244896, 28348.561224489797, 28258.377551020407, 28274.35714285714, 28046.54081632653, 28039.84693877551, 28163.51020408163, 27994.418367346938, 27789.84693877551, 27786.724489795917, 27765.316326530614, 27687.19387755102, 27616.275510204083, 27594.632653061224, 27495.30612244898, 27333.602040816328, 27321.918367346938, 27214.5, 27084.84693877551, 27027.663265306124, 26885.01020408163, 26820.724489795917, 26843.80612244898, 26775.897959183672, 26582.755102040817, 26468.01020408163, 26509.448979591838, 26347.38775510204, 26246.70408163265, 26076.19387755102, 25936.020408163266, 25814.45918367347, 25805.5, 25693.73469387755, 25635.724489795917, 25643.23469387755, 25456.20408163265, 25285.0, 25352.867346938776, 25215.285714285714, 25146.591836734693, 25130.948979591838, 24985.98979591837, 24843.122448979593, 24791.102040816328, 24754.530612244896, 24654.520408163266, 24542.73469387755, 24495.04081632653, 24487.877551020407, 24404.979591836734, 24295.23469387755, 24306.714285714286, 24226.5, 24179.785714285714, 24306.724489795917, 24099.04081632653, 23980.316326530614, 23929.95918367347, 23730.377551020407, 23668.867346938776, 23663.04081632653, 23568.80612244898, 23642.928571428572, 23677.14285714286, 23708.030612244896, 23678.214285714286, 23698.755102040817, 23720.5, 23686.683673469386, 23594.79591836735, 23615.724489795917, 23637.581632653062, 23593.775510204083, 23561.724489795917, 23602.79591836735, 23572.61224489796, 23665.64285714286, 23609.5, 23745.73469387755, 23638.469387755104, 23652.622448979593, 23733.377551020407, 23601.816326530614, 23709.95918367347, 23671.938775510203, 23769.255102040817, 23770.23469387755, 23820.448979591838, 23872.714285714286, 23844.561224489797, 23855.663265306124, 23952.173469387755, 24046.571428571428, 24066.367346938776, 24019.79591836735, 24093.571428571428, 24201.469387755104, 24149.64285714286, 24295.95918367347, 24328.061224489797, 24342.15306122449, 24263.551020408162, 24326.561224489797, 24392.336734693876, 24424.867346938776, 24423.285714285714, 24604.20408163265, 24561.34693877551, 24681.418367346938, 24709.530612244896, 24809.714285714286, 24964.95918367347, 24936.84693877551, 25144.0, 25134.581632653062, 25251.938775510203, 25463.418367346938, 25449.51020408163, 25539.30612244898, 25647.979591836734, 25671.918367346938, 25948.15306122449, 25938.316326530614, 26008.01020408163, 25879.744897959183, 25930.867346938776, 25914.0, 25994.908163265307, 25986.61224489796, 25921.908163265307, 25880.38775510204, 25863.673469387755, 25875.29591836735, 25818.632653061224, 25923.54081632653, 25936.091836734693, 25999.244897959183, 26021.071428571428, 26009.14285714286, 25969.214285714286, 25993.01020408163, 26054.897959183672, 26051.479591836734, 26117.714285714286, 26112.663265306124, 26145.11224489796, 26081.530612244896, 26133.316326530614, 25987.34693877551, 25937.54081632653, 25816.01020408163, 25827.755102040817, 25816.622448979593, 25921.061224489797, 25936.775510204083, 25893.367346938776, 25838.64285714286, 25916.673469387755, 25835.755102040817, 25762.79591836735, 25805.908163265307, 25872.938775510203, 25784.95918367347, 25777.377551020407, 25778.030612244896, 25684.418367346938, 25657.45918367347, 25643.80612244898, 25724.663265306124, 25678.581632653062, 25573.35714285714, 25522.48979591837, 25438.132653061224, 25530.30612244898, 25451.622448979593, 25501.183673469386, 25403.591836734693, 25445.34693877551, 25249.428571428572, 25292.020408163266, 25163.275510204083, 25219.448979591838, 25228.928571428572, 25187.26530612245, 25009.51020408163, 25012.867346938776, 24963.367346938776, 24965.132653061224, 25032.244897959183, 24837.29591836735, 24733.826530612245, 24726.35714285714, 24605.51020408163, 24638.438775510203, 24518.448979591838, 24446.34693877551, 24473.244897959183, 24386.683673469386, 24281.551020408162, 24220.214285714286, 24227.673469387755, 24137.408163265307, 24145.61224489796, 24068.98979591837, 24080.65306122449, 23838.0, 23783.20408163265, 23869.30612244898, 23785.877551020407, 23709.836734693876, 23704.673469387755, 23696.30612244898, 23523.45918367347, 23475.561224489797, 23415.54081632653, 23327.051020408162, 23326.397959183672, 23354.26530612245, 23138.081632653062, 23120.020408163266, 23100.775510204083, 22950.173469387755, 22903.571428571428, 22895.15306122449, 22820.04081632653, 22736.51020408163, 22625.29591836735, 22687.5, 22597.979591836734, 22531.326530612245, 22484.561224489797, 22550.19387755102, 22479.224489795917, 22433.255102040817, 22269.775510204083, 22051.98979591837, 21983.897959183672, 21933.183673469386, 21822.520408163266, 21831.316326530614, 21735.030612244896, 21653.755102040817, 21636.683673469386, 21628.918367346938, 21479.64285714286, 21433.081632653062, 21354.26530612245, 21255.23469387755, 21177.102040816328, 21186.80612244898, 21072.285714285714, 21047.479591836734, 20957.520408163266, 20912.755102040817, 20813.214285714286, 20794.70408163265, 20741.35714285714, 20707.26530612245, 20568.65306122449, 20525.744897959183, 20503.0, 20382.479591836734, 20364.122448979593, 20319.336734693876, 20191.448979591838, 20167.84693877551, 20086.785714285714, 20004.173469387755, 19987.20408163265, 19951.01020408163, 19873.591836734693, 19792.979591836734, 19710.469387755104, 19658.64285714286, 19473.163265306124, 19428.88775510204, 19436.316326530614, 19363.061224489797, 19302.571428571428, 19223.775510204083, 19127.051020408162, 19197.326530612245, 19028.51020408163, 18937.867346938776, 18845.591836734693, 18811.071428571428, 18781.38775510204, 18711.724489795917, 18624.95918367347, 18586.408163265307, 18514.173469387755, 18425.88775510204, 18399.561224489797, 18284.479591836734, 18320.061224489797, 18168.836734693876, 17972.602040816328, 17731.520408163266, 17431.428571428572, 17301.183673469386, 17272.714285714286, 17389.224489795917, 17490.336734693876, 17494.5, 17450.01020408163, 17346.867346938776, 17267.244897959183, 17232.70408163265, 17217.73469387755, 17155.15306122449, 17025.15306122449, 17027.020408163266, 16975.785714285714, 16863.744897959183, 16800.336734693876, 16747.285714285714, 16664.64285714286, 16597.102040816328, 16563.30612244898, 16453.908163265307, 16402.122448979593, 16401.081632653062, 16345.112244897959, 16387.183673469386, 16329.438775510203, 16292.42857142857, 16239.673469387755, 16209.836734693878, 16069.224489795919, 16011.275510204081, 15872.724489795919, 15785.091836734693, 15717.234693877552, 15582.5, 15502.867346938776, 15468.918367346938, 15348.92857142857, 15274.581632653062, 15246.591836734693, 15130.591836734693, 15074.540816326531, 14953.602040816326, 14924.948979591836, 14894.15306122449, 14811.816326530612, 14722.5, 14727.183673469388, 14656.908163265307, 14593.591836734693, 14497.336734693878, 14463.19387755102, 14433.275510204081, 14363.0, 14278.816326530612, 14261.020408163266, 14230.367346938776, 14170.989795918367, 14153.336734693878, 14015.132653061224, 14029.744897959185, 13932.581632653062, 13879.102040816326, 13829.887755102041, 13797.540816326531, 13740.387755102041, 13710.663265306122, 13666.336734693878, 13618.357142857143, 13557.367346938776, 13478.326530612245, 13452.510204081633, 13427.275510204081, 13424.387755102041, 13327.061224489797, 13296.397959183674, 13308.183673469388, 13293.336734693878, 13226.224489795919, 13213.581632653062, 13169.57142857143, 13060.765306122448, 13040.387755102041, 13015.5, 12955.69387755102, 12938.112244897959, 12937.15306122449, 12887.918367346938, 12826.448979591836, 12813.877551020409, 12781.30612244898, 12801.69387755102, 12729.673469387755, 12639.724489795919, 12662.459183673469, 12632.591836734693, 12633.42857142857, 12588.459183673469, 12624.612244897959, 12562.010204081633, 12524.704081632653, 12466.969387755102, 12383.836734693878, 12391.591836734693, 12381.867346938776, 12383.265306122448, 12358.326530612245, 12364.275510204081, 12290.84693877551, 12254.602040816326, 12200.69387755102, 12194.30612244898, 12188.5, 12168.234693877552, 12182.887755102041, 12126.765306122448, 12105.683673469388, 12112.948979591836, 12063.948979591836, 12010.785714285714, 12025.295918367347, 11991.5, 12024.69387755102, 11940.295918367347, 11903.19387755102, 11917.540816326531, 11923.30612244898, 11877.948979591836, 11857.80612244898, 11838.459183673469, 11800.255102040815, 11832.0, 11780.418367346938, 11755.908163265307, 11712.816326530612, 11705.642857142857, 11699.92857142857, 11687.897959183674, 11653.408163265307, 11554.040816326531, 11560.612244897959, 11525.42857142857, 11556.897959183674, 11511.581632653062, 11504.34693877551, 11445.561224489797, 11480.65306122449, 11457.142857142857, 11422.265306122448, 11420.510204081633, 11347.081632653062, 11330.755102040815, 11358.908163265307, 11302.367346938776, 11268.57142857143, 11300.92857142857, 11242.15306122449, 11228.418367346938, 11199.908163265307, 11161.0, 11101.30612244898, 11092.061224489797, 11149.673469387755, 11098.15306122449, 11049.989795918367, 10989.367346938776, 11016.897959183674, 11033.091836734693, 10986.795918367347, 10984.540816326531, 10968.469387755102, 10920.408163265307, 10899.959183673469, 10872.336734693878, 10852.520408163266, 10841.367346938776, 10842.122448979591, 10812.989795918367, 10820.377551020409, 10745.448979591836, 10764.540816326531, 10771.80612244898, 10739.897959183674, 10662.204081632653, 10631.683673469388, 10577.469387755102, 10536.19387755102, 10555.244897959185, 10502.316326530612, 10503.673469387755, 10455.918367346938, 10453.285714285714, 10377.581632653062, 10397.673469387755, 10379.397959183674, 10360.826530612245, 10348.214285714286, 10320.418367346938, 10262.959183673469, 10188.673469387755, 10159.959183673469, 10168.081632653062, 10127.19387755102, 10121.234693877552, 10098.112244897959, 10077.061224489797, 10012.19387755102, 9963.826530612245, 9940.714285714286, 9943.387755102041, 9920.040816326531, 9849.65306122449, 9868.275510204081, 9814.591836734693, 9703.0, 9706.714285714286, 9695.683673469388, 9688.122448979591, 9669.489795918367, 9653.765306122448, 9595.408163265307, 9549.622448979591, 9503.397959183674, 9485.061224489797, 9454.418367346938, 9457.0, 9409.510204081633, 9360.42857142857, 9343.969387755102, 9326.632653061224, 9283.867346938776, 9258.377551020409, 9198.19387755102, 9125.265306122448, 9138.663265306122, 9144.19387755102, 9133.112244897959, 9094.724489795919, 9043.948979591836, 9035.010204081633, 9001.581632653062, 8979.42857142857, 8948.602040816326, 8948.5, 8903.632653061224, 8852.632653061224, 8775.948979591836, 8780.418367346938, 8731.663265306122, 8706.959183673469, 8688.0, 8618.979591836734, 8616.438775510203, 8572.520408163266, 8545.42857142857, 8498.65306122449, 8473.867346938776, 8464.948979591836, 8445.84693877551, 8388.989795918367, 8353.959183673469, 8337.918367346938, 8311.183673469388, 8265.591836734693, 8240.19387755102, 8194.642857142857, 8201.561224489797, 8164.4795918367345, 8124.714285714285, 8100.7040816326535, 8049.836734693878, 8033.734693877551, 7995.622448979592, 7961.071428571428, 7911.857142857143, 7903.2040816326535, 7852.0204081632655, 7834.785714285715, 7815.0, 7769.622448979592, 7781.15306122449, 7730.683673469388, 7668.765306122449, 7643.0204081632655, 7642.867346938776, 7616.5, 7559.336734693878, 7548.265306122449, 7519.030612244898, 7489.571428571428, 7442.173469387755, 7407.877551020408, 7381.010204081633, 7349.765306122449, 7319.265306122449, 7305.826530612245, 7282.306122448979, 7239.122448979592, 7195.632653061224, 7158.908163265306, 7172.285714285715, 7143.102040816327, 7126.336734693878, 7100.316326530612, 7040.102040816327, 7015.622448979592, 6994.367346938776, 6970.928571428572, 6929.867346938776, 6889.122448979592, 6835.918367346939, 6853.326530612245, 6810.193877551021, 6765.091836734694, 6767.367346938776, 6719.744897959184, 6682.438775510204, 6688.561224489796, 6642.0, 6631.928571428572, 6605.5, 6593.102040816327, 6578.683673469388, 6542.469387755102, 6497.408163265306, 6490.4795918367345, 6457.1122448979595, 6426.908163265306, 6400.530612244898, 6351.724489795918, 6340.244897959184, 6314.551020408163, 6296.122448979592, 6283.755102040816, 6266.418367346939, 6239.367346938776, 6211.734693877551, 6168.336734693878, 6162.775510204082, 6132.724489795918, 6104.173469387755, 6089.928571428572, 6037.622448979592, 6023.9795918367345, 5993.714285714285, 5974.244897959184, 5947.7040816326535, 5921.714285714285, 5906.051020408163, 5865.244897959184, 5861.877551020408, 5821.030612244898, 5809.65306122449, 5799.316326530612, 5778.714285714285, 5739.2040816326535, 5724.989795918367, 5695.4795918367345, 5676.724489795918, 5655.84693877551, 5642.816326530612, 5634.285714285715, 5593.581632653061, 5578.551020408163, 5555.010204081633, 5545.693877551021, 5536.806122448979, 5499.3877551020405, 5467.367346938776, 5442.081632653061, 5435.683673469388, 5399.561224489796, 5396.510204081633, 5377.1122448979595, 5357.408163265306, 5327.642857142857, 5312.316326530612, 5311.244897959184, 5276.867346938776, 5257.5204081632655, 5249.326530612245, 5226.214285714285, 5185.959183673469, 5163.959183673469, 5155.040816326531, 5138.255102040816, 5121.938775510204, 5101.193877551021, 5095.163265306122, 5059.551020408163, 5045.469387755102, 5026.15306122449, 5013.5204081632655, 5011.724489795918, 5001.030612244898, 4957.255102040816, 4931.602040816327, 4945.0204081632655, 4926.581632653061, 4912.163265306122, 4889.744897959184, 4874.7959183673465, 4857.183673469388, 4844.234693877551, 4827.102040816327, 4809.071428571428, 4789.9795918367345, 4774.744897959184, 4750.836734693878, 4745.285714285715, 4729.224489795918, 4717.673469387755, 4686.091836734694, 4685.489795918367, 4658.571428571428, 4640.989795918367, 4643.459183673469, 4613.826530612245, 4595.459183673469, 4574.357142857143, 4563.571428571428, 4555.551020408163, 4514.897959183673, 4495.714285714285, 4446.34693877551, 4468.642857142857, 4483.948979591837, 4469.6122448979595, 4446.2959183673465, 4429.744897959184, 4388.826530612245, 4327.1122448979595, 4276.255102040816, 4338.489795918367, 4336.265306122449, 4329.234693877551, 4321.7959183673465, 4313.561224489796, 4281.234693877551, 4253.173469387755, 4224.581632653061, 4169.724489795918, 4176.438775510204, 4192.897959183673, 4168.091836734694, 4176.673469387755, 4166.897959183673, 4162.84693877551, 4132.642857142857, 4108.336734693878, 4059.173469387755, 4016.8979591836733, 4053.030612244898, 4057.9489795918366, 4034.591836734694, 4029.908163265306, 3993.3469387755104, 3947.8979591836733, 3988.734693877551, 3931.0408163265306, 3859.8673469387754, 3819.581632653061, 3820.9285714285716, 3842.326530612245, 3818.8061224489797, 3890.9591836734694, 3899.326530612245, 3875.4795918367345, 3892.7755102040815, 3870.234693877551, 3854.816326530612, 3823.8367346938776, 3771.234693877551, 3700.622448979592, 3733.1632653061224, 3772.265306122449, 3746.061224489796, 3675.714285714286, 3687.5714285714284, 3732.0408163265306, 3727.1428571428573, 3736.326530612245, 3703.908163265306, 3699.8061224489797, 3686.173469387755, 3649.377551020408, 3632.1530612244896, 3621.9795918367345, 3629.061224489796, 3623.2244897959185, 3572.5714285714284, 3573.765306122449, 3502.214285714286, 3512.9285714285716, 3573.2551020408164, 3551.581632653061, 3547.6020408163267, 3540.1632653061224, 3507.5510204081634, 3444.1938775510203, 3467.408163265306, 3480.4591836734694, 3460.173469387755, 3388.795918367347, 3432.183673469388, 3445.3367346938776, 3426.8061224489797, 3437.3979591836733, 3412.5714285714284, 3372.6326530612246, 3370.5714285714284, 3398.6326530612246, 3375.6632653061224, 3379.612244897959, 3363.918367346939, 3351.2551020408164, 3326.3673469387754, 3321.438775510204, 3311.2551020408164, 3302.5714285714284, 3295.1938775510203, 3271.8061224489797, 3254.908163265306, 3231.122448979592, 3221.561224489796, 3223.4285714285716, 3214.0204081632655, 3201.5510204081634, 3187.6938775510203, 3177.326530612245, 3171.734693877551, 3163.6428571428573, 3145.5, 3152.4795918367345, 3126.7244897959185, 3098.9591836734694, 3083.5510204081634, 3093.1530612244896, 3074.826530612245, 3071.714285714286, 3051.785714285714, 3050.234693877551, 3015.204081632653, 2987.3673469387754, 2996.816326530612, 3000.7551020408164, 2982.3571428571427, 2967.091836734694, 2935.622448979592, 2938.173469387755, 2932.938775510204, 2921.9795918367345, 2896.469387755102, 2837.795918367347, 2794.9897959183672, 2781.1530612244896, 2817.826530612245, 2830.7551020408164, 2808.8061224489797, 2823.0408163265306, 2823.0204081632655, 2813.4795918367345, 2790.8061224489797, 2786.1530612244896, 2777.969387755102, 2736.785714285714, 2712.7755102040815, 2725.877551020408, 2686.908163265306, 2601.1020408163267, 2655.4591836734694, 2678.5, 2662.9795918367345, 2661.826530612245, 2655.6326530612246, 2647.295918367347, 2644.7448979591836, 2643.2448979591836, 2632.204081632653, 2614.2448979591836, 2604.6632653061224, 2596.0408163265306, 2591.887755102041, 2567.918367346939, 2545.785714285714, 2528.0510204081634, 2507.8061224489797, 2530.877551020408, 2527.1530612244896, 2500.316326530612, 2478.1938775510203, 2449.969387755102, 2464.214285714286, 2469.7448979591836, 2467.214285714286, 2455.0, 2447.8367346938776, 2443.6020408163267, 2425.2448979591836, 2412.6020408163267, 2407.081632653061, 2382.8979591836733, 2395.887755102041, 2395.3061224489797, 2379.8061224489797, 2366.091836734694, 2360.5510204081634, 2344.387755102041, 2337.3979591836733, 2340.7551020408164, 2337.673469387755, 2313.204081632653, 2298.030612244898, 2267.4489795918366, 2234.183673469388, 2246.1020408163267, 2276.734693877551, 2277.765306122449, 2256.2244897959185, 2247.4285714285716, 2239.918367346939, 2235.714285714286, 2231.316326530612, 2219.377551020408, 2211.938775510204, 2205.091836734694, 2186.265306122449, 2178.4591836734694, 2135.091836734694, 2142.8673469387754, 2151.9591836734694, 2146.091836734694, 2137.112244897959, 2131.173469387755, 2124.091836734694, 2099.2755102040815, 2071.295918367347, 2093.683673469388, 2094.1632653061224, 2098.3673469387754, 2095.918367346939, 2084.673469387755, 2083.2244897959185, 2068.8061224489797, 2066.1020408163267, 2059.3979591836733, 2051.8979591836733, 2044.8163265306123, 2035.2142857142858, 2025.9285714285713, 2028.5408163265306, 2014.7448979591836, 2007.1020408163265, 1981.857142857143, 1975.0714285714287, 1981.3469387755101, 1972.6224489795918, 1975.295918367347, 1963.2448979591836, 1943.3367346938776, 1938.408163265306, 1953.9285714285713, 1942.6632653061224, 1932.6530612244899, 1937.5510204081634, 1927.2857142857142, 1920.295918367347, 1911.1530612244899, 1914.1122448979593, 1912.2857142857142, 1908.3367346938776, 1901.1326530612246, 1888.469387755102, 1885.1836734693877, 1876.7755102040817, 1865.2142857142858, 1868.2448979591836, 1861.969387755102, 1855.8367346938776, 1853.6734693877552, 1845.5714285714287, 1837.3979591836735, 1823.5102040816328, 1805.9795918367347, 1799.4897959183672, 1813.8469387755101, 1808.857142857143, 1807.938775510204, 1802.2755102040817, 1790.642857142857, 1787.9591836734694, 1782.3673469387754, 1776.0408163265306, 1772.4285714285713, 1747.9897959183672, 1747.5102040816328, 1743.0714285714287, 1743.4285714285713, 1739.3265306122448, 1727.530612244898, 1727.5510204081634, 1721.4183673469388, 1719.3673469387754, 1711.1020408163265, 1698.969387755102, 1697.357142857143, 1683.142857142857, 1681.3979591836735, 1671.8265306122448, 1660.8061224489795, 1665.1224489795918, 1660.1326530612246, 1658.734693877551, 1649.7551020408164, 1643.8979591836735, 1638.3061224489795, 1635.1122448979593, 1634.908163265306, 1623.765306122449, 1619.765306122449, 1617.642857142857, 1613.1938775510205, 1601.8061224489795, 1587.5714285714287, 1578.5, 1579.9285714285713, 1579.2857142857142, 1571.734693877551, 1563.8979591836735, 1560.0, 1558.1122448979593, 1547.561224489796, 1540.5408163265306, 1532.8979591836735, 1530.3163265306123, 1525.8673469387754, 1523.7448979591836, 1515.857142857143, 1512.704081632653, 1508.7755102040817, 1506.4183673469388, 1503.3367346938776, 1496.5, 1489.8469387755101, 1488.530612244898, 1482.5102040816328, 1475.5510204081634, 1473.5510204081634, 1472.5204081632653, 1468.204081632653, 1453.9897959183672, 1447.4285714285713, 1445.469387755102, 1443.9183673469388, 1433.5408163265306, 1434.4591836734694, 1430.4591836734694, 1426.7857142857142, 1416.3673469387754, 1415.704081632653, 1409.6326530612246, 1409.561224489796, 1402.908163265306, 1394.3163265306123, 1389.357142857143, 1387.7857142857142, 1390.6326530612246, 1382.3061224489795, 1369.1632653061224, 1366.3265306122448, 1366.4285714285713, 1364.969387755102, 1351.2448979591836, 1353.0408163265306, 1350.7551020408164, 1348.438775510204, 1343.9795918367347, 1337.295918367347, 1337.765306122449, 1331.3469387755101, 1330.3265306122448, 1315.9795918367347, 1319.0102040816328, 1314.265306122449, 1311.6530612244899, 1303.2857142857142, 1299.234693877551, 1292.8265306122448, 1289.938775510204, 1289.357142857143, 1281.1326530612246, 1282.2448979591836, 1280.969387755102, 1271.9897959183672, 1266.3979591836735, 1269.9285714285713, 1259.5816326530612, 1259.4285714285713, 1258.3979591836735, 1252.0408163265306, 1247.9591836734694, 1247.8265306122448, 1240.469387755102, 1231.8061224489795, 1233.0714285714287, 1231.1734693877552, 1228.908163265306, 1222.8061224489795, 1222.2244897959183, 1215.591836734694, 1213.295918367347, 1207.9795918367347, 1201.0714285714287, 1203.9795918367347, 1201.8877551020407, 1193.6632653061224, 1192.4489795918366, 1189.5816326530612, 1185.9591836734694, 1182.0, 1177.8469387755101, 1170.061224489796, 1166.765306122449, 1173.091836734694, 1160.2142857142858, 1157.1224489795918, 1160.5714285714287, 1154.8877551020407, 1146.795918367347, 1143.0102040816328, 1139.561224489796]
  in  "t0 position":u32=3
  out "?":dbl[](graph)
  in  "?":bool
  in  "# of Sets":i32
  out "Current Set":u32=24
  in  "#Ground per set":u32=3
  in  "Timepoints":dbl[](array[numeric])=[200.0, 100.0, 300.0, 400.0, 500.0]
  in  "File Path":path
  in  "File Name":string
  in  "Ground State\nSubstract?":bool
  in  "?":enum16{"FOCUS", "WINSPEC"}(ring)
  in  "Center Wavelength":dbl format="%.2f"
  in  "?":bool
  out "?":dbl[](graph)
  in  "?":bool
  in  "Save to a File":bool
  out "Current Wavelength":string
  in  "Grating Number":i16=1 min=1 max=100 step=1
  in  "Grating Speed":dbl=2000.0 min=1.0 step=1.0 format="%.1f"
  in  "Start Wavelength":dbl format="%.2f"
  in  "End Wavelength":dbl=700.0 format="%.2f"
  in  "Increment Wavelength":dbl=50.0 format="%.2f"
  in  "Turret Number":i16=1
  in  "Spectrograph error in":errorcluster
  out "Spectrograph \nerror out":errorcluster
  in  "File Path":path
  in  "File Name":string
  out "Spectrometer\nhandle":u32
  in  "Mirror Number":i16=1 min=1 max=4 step=1
  in  "Position":i16=1 min=1 max=2 step=1
  in  "?":bool
  out "Ready to Run":bool
  in  "Number of Images":u32=200 min=1 step=1
  # "kHz"
  # "ms"
  # "ms"
  # "Triggering"
  # "Seconds"
  # "Temperature"
  # "°C"
  # "ADC"
  # "-3 = Slowest speed\n-2 = Fastest speed\n-1 =Default speed or enter speed in kHz"
  # "Shutter"
  # "Shutter Times"
  # "ms"
  # "Cleans / Clears"
  # "Custom Chip and Timing"
  # "Kinetics Timing"
  # "Logic Output"
  # "Region Of Interest"
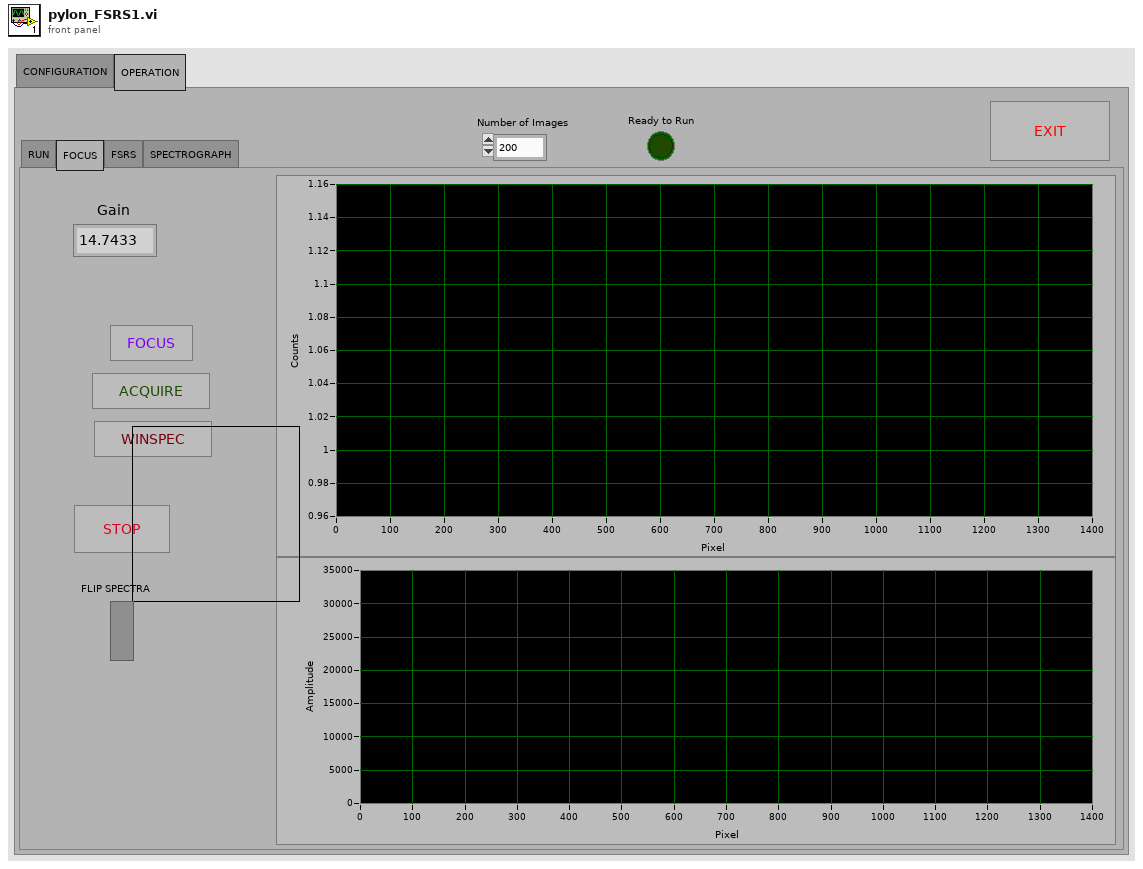
[diagram p1: front panel]
types:
  T1 = enum32{"Trigger", "Temperature", "ADC", "Shutter", "Cleans/Clears", "Custom", "Logic Out", "ROI"}
  T2 = enum8{"Enabled", "Disabled", "Disabled and Grayed Out"}
  T3 = cluster{"Camera Number":i32, "ROI Number":i32, "X Start":i32, "X End":i32, "X Bin":i32, "Y Start":i32, "Y End":i32, "Y Bin":i32}
  T4 = cluster{"Pre Y":u32, "Post Y":u32, "Active Y":u32, "Pre X":u32, "Post X":u32, "Active X":u32, "Custom Chip Enabled":bool, "Vertical Timing Index":u32}
  T5 = cluster{"Exposure":dbl, "Collection Mode":u32, "Timing Mode":u32, "Trigger Edge":u32, "Temperature":dbl}
  T6 = cluster{"ADC Speed":i32, "ADC Gain":i32, "ADC Offset":i32, "Readout Port":i32, "Num Cleans":u32, "Num Strips per Clean":u32, "Mini Block Size":u32, "Num Min Blocks":u32, "Continous Cleans":bool, "Skip Serial Reg Clean":bool}
  T7 = cluster{"Shutter State":u16, "Open Comp Time ":u32, "Close Comp Time":u32, "Logic Out Setting":u32, "Logic Out Invert":bool}
  T8 = cluster{"acquire focus mode":u32, "Exposure Time (s)":dbl, i32, "Software accumulation":u32}
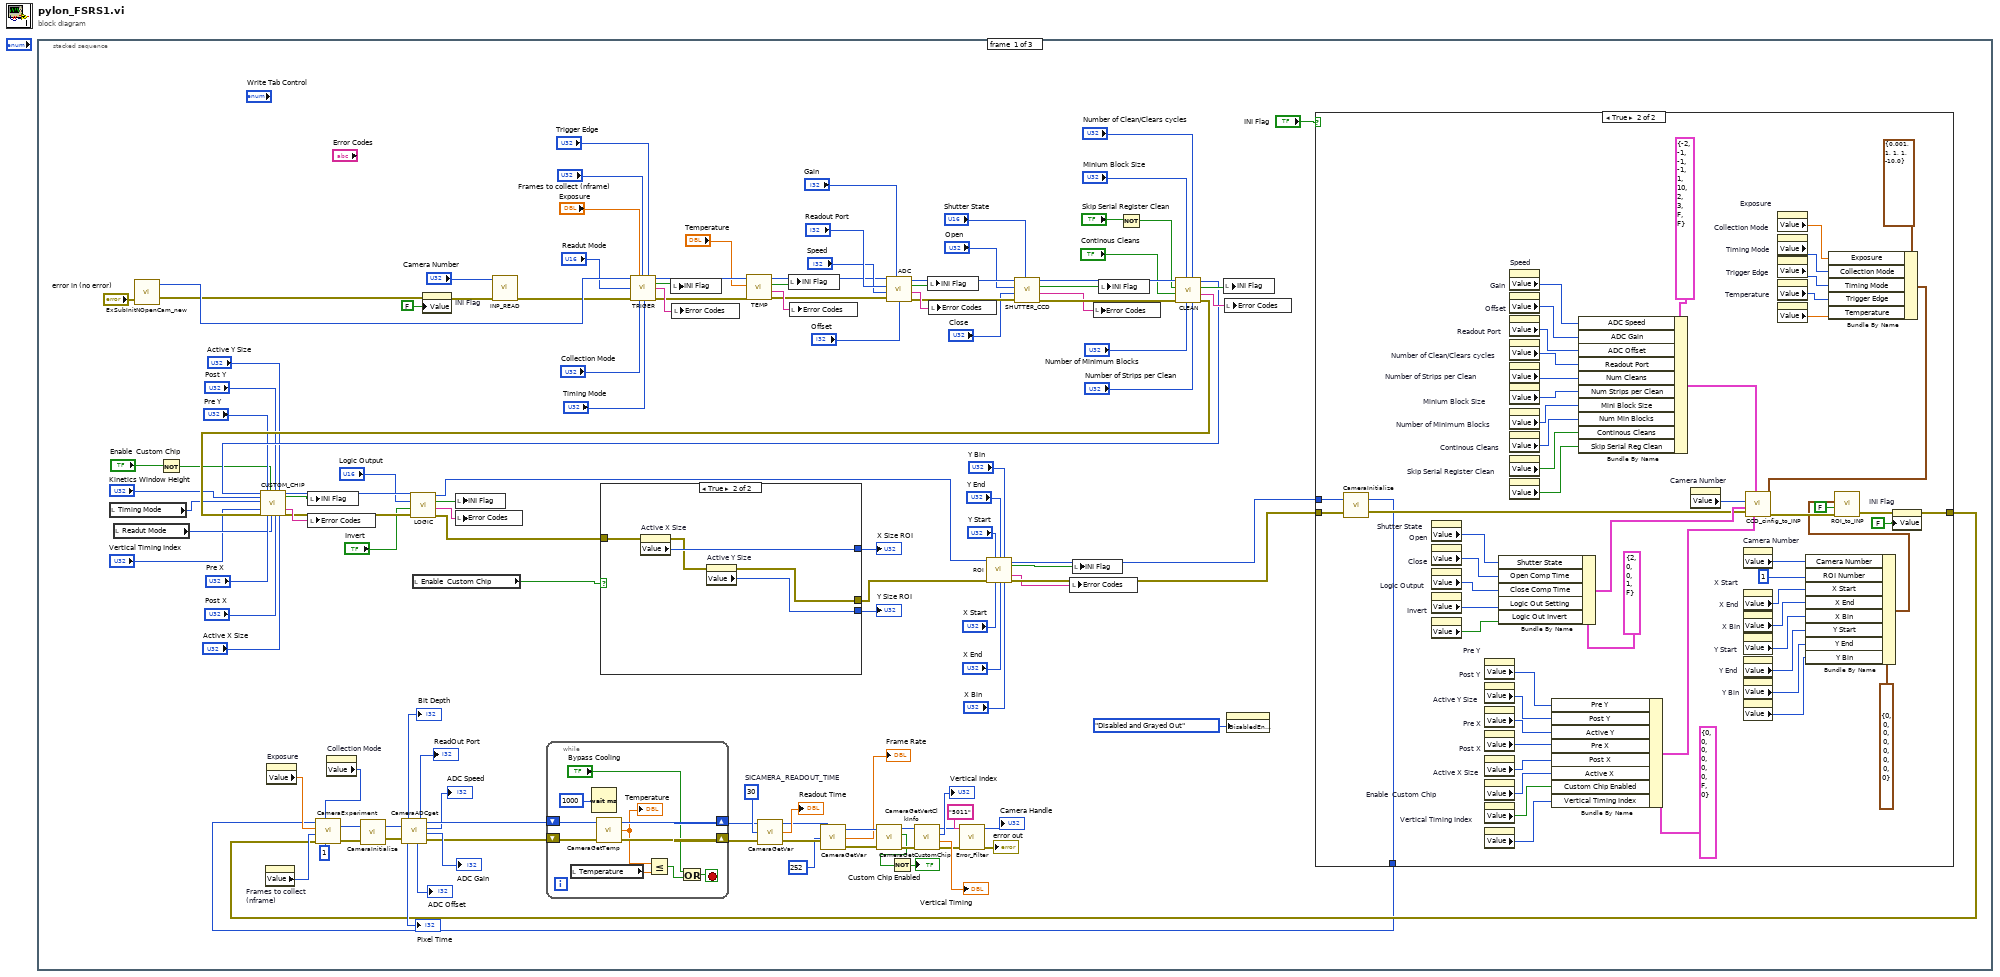
[diagram p0: block diagram]
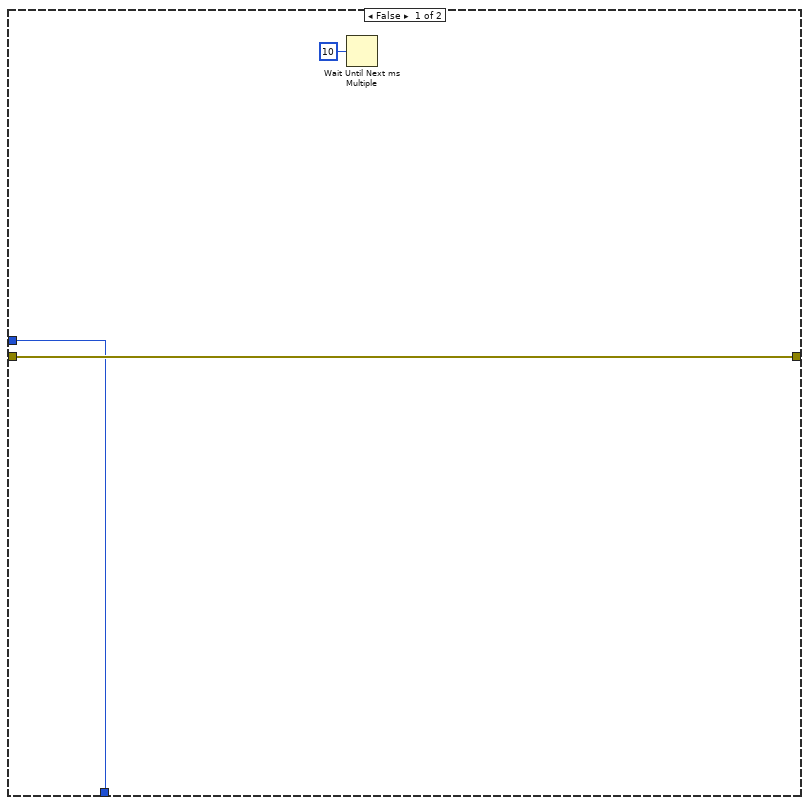
[diagram p2: hidden frame]
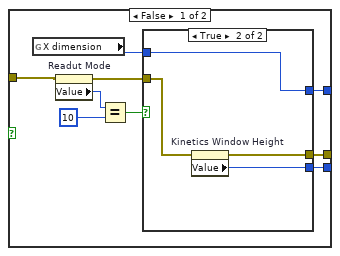
[diagram p3: hidden frame]
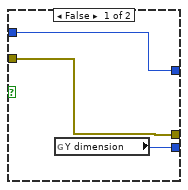
[diagram p4: hidden frame]
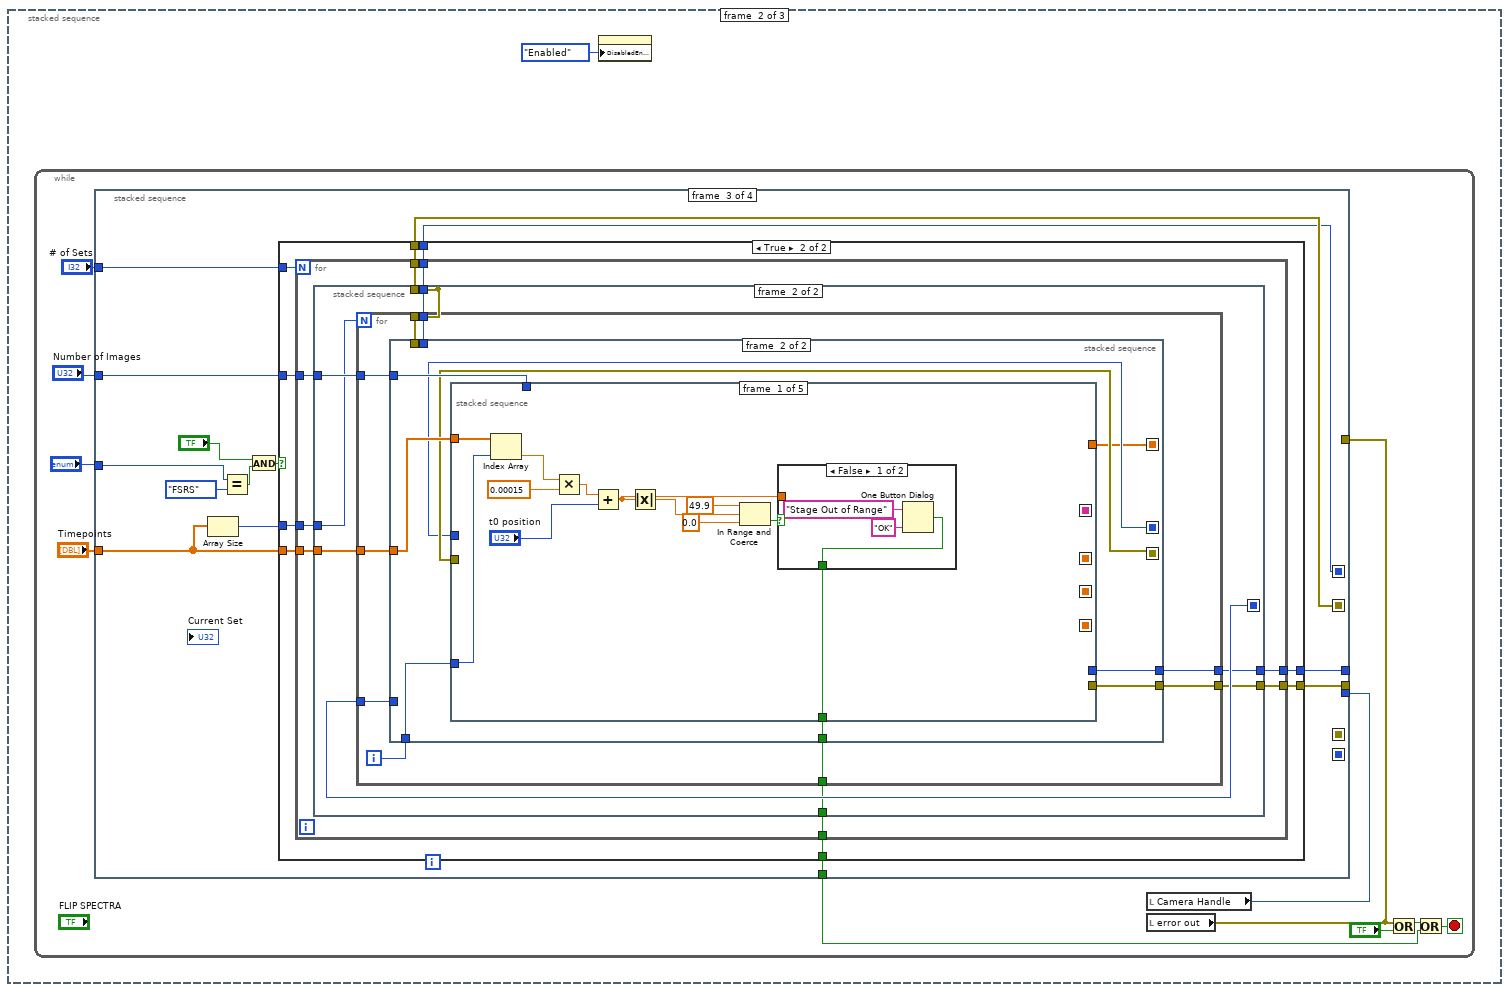
[diagram p5: hidden frame]
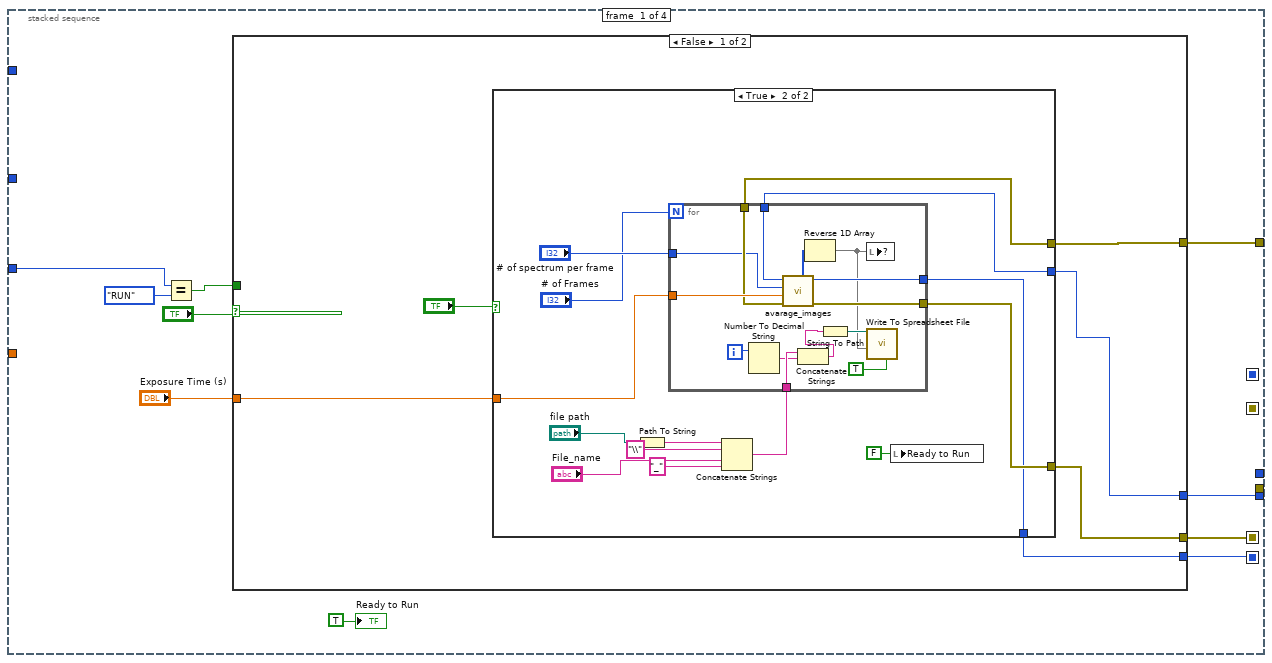
[diagram p6: hidden frame]
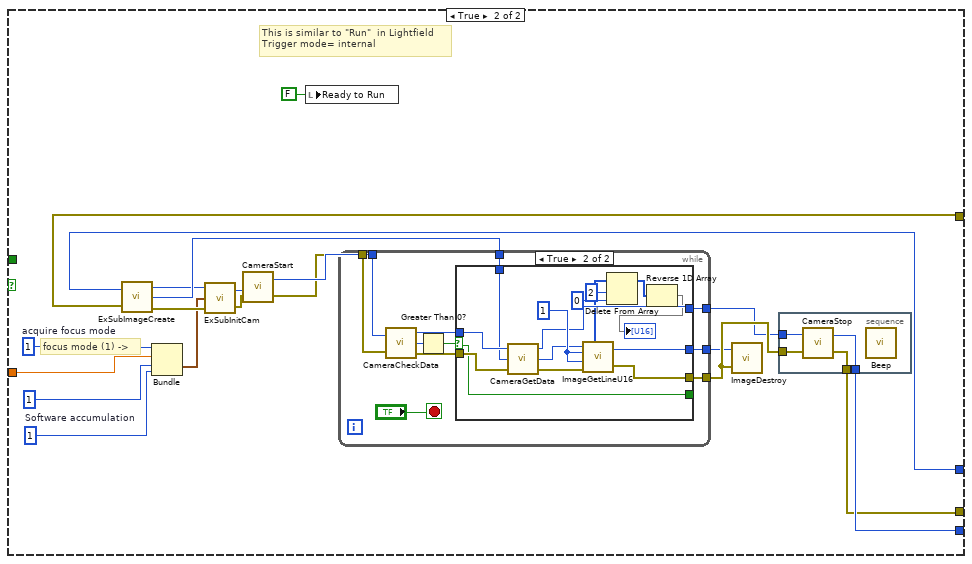
[diagram p8: hidden frame]
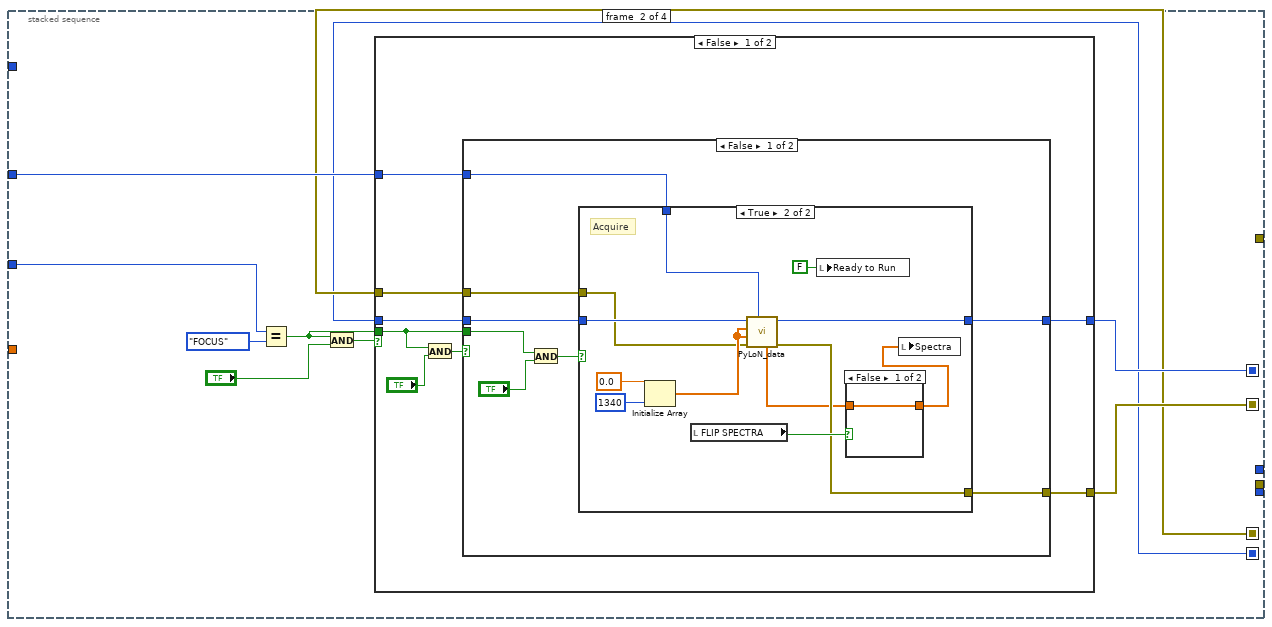
[diagram p10: hidden frame]
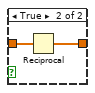
[diagram p12: hidden frame]
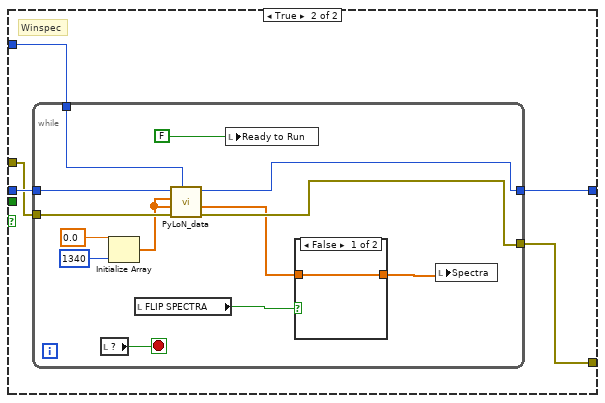
[diagram p13: hidden frame]
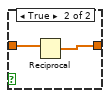
[diagram p14: hidden frame]
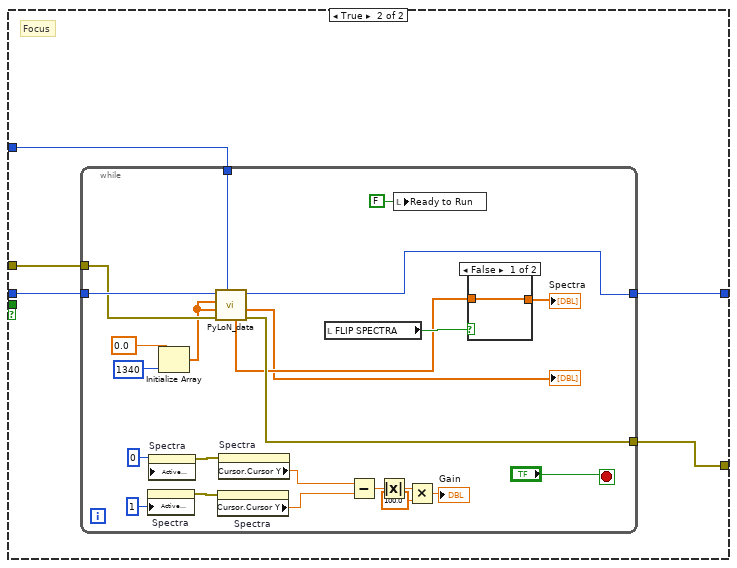
[diagram p15: hidden frame]
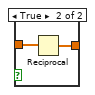
[diagram p16: hidden frame]
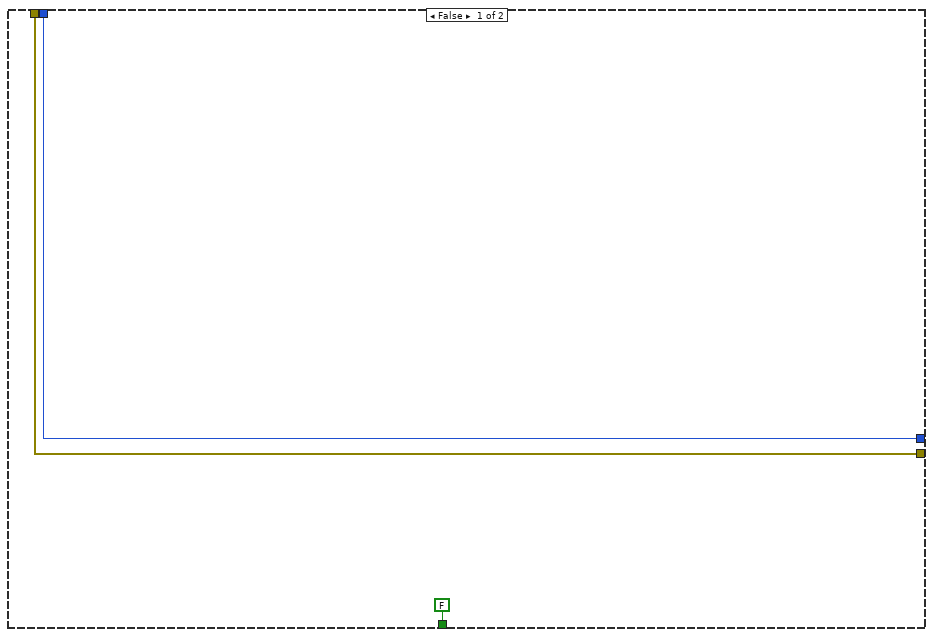
[diagram p17: hidden frame]
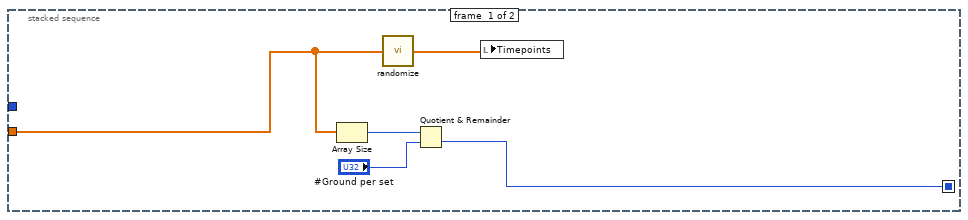
[diagram p18: hidden frame]
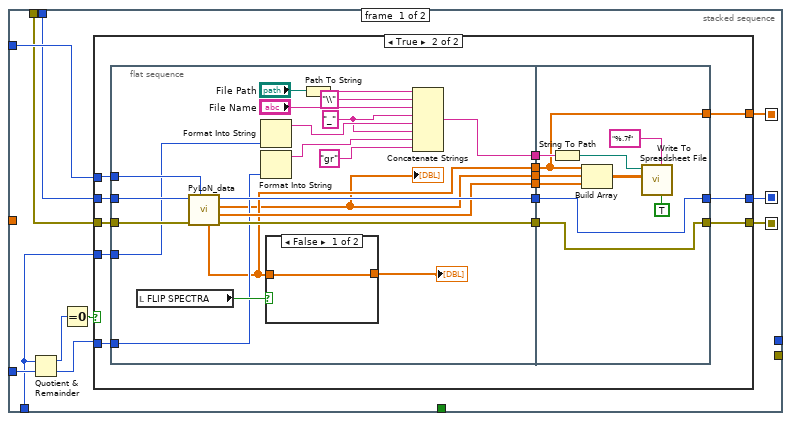
[diagram p19: hidden frame]
diagram:
  n1 = stacked-sequence {
    frame #0 {
      w40 = 30  # SICAMERA_READOUT_TIME
      n2 = local read "Timing Mode"() -> (w70:u32)
      n3 = local read "Readut Mode"() -> (w71:u16)
      n4 = call "ExSubInitNOpenCam_new.vi"("error in (no error)"="error in (no error)") -> ("Camera Handle"=w122:u32, "error out"=w1:errorcluster)  [unwired: 1 in]
      n5 = Not(x="Enable  Custom Chip") -> (.not. x?=w6:bool)
      n6 = property on="Frames to collect (nframe)" class="DigNum (strict)"() -> ("Value"=w19:u32)  [unwired: 2 in, 2 out]
      n7 = property on="Exposure" class="DigNum (strict)"() -> ("Value"=w22:dbl)  [unwired: 2 in, 2 out]
      n8 = property on="Collection Mode" class="Ring (strict)"() -> ("Value"=w17:u32)  [unwired: 2 in, 2 out]
      n9 = local read "Enable  Custom Chip"() -> (w61:bool)
      n10 = property on="INI Flag" class="Bool (strict)"(error in=w1, "Value"=FALSE) -> (error out=w107:errorcluster)  [unwired: 1 in, 1 out]
      n11 = call "INP_READ.vi"("error in (no error)"=w107, "Camera Number"="Camera Number") -> ("error out"=w106:errorcluster)  [unwired: 4 in, 5 out]
      n12 = call "TRIGER.vi"("Camera Handle"=w122, "Exposure (sec)"="Exposure", "Number of frams"="Frames to collect (nframe)", "Trigger Edge"="Trigger Edge", "ReadOut Mode"="Readut Mode", "error out"=w106, "Acquire / Focus Flag"="Collection Mode", "Timing Mode"="Timing Mode") -> ("Camera Handle"=w113:u32, "INI Flag"=w115:bool, "String"=w114:string, "error out"=w112:errorcluster)  [unwired: 4 in]
      n13 = local write "INI Flag"(w115) -> ()
      n14 = local write "Error Codes"(w114) -> ()
      n15 = call "TEMP.vi"("error in (no error)"=w112, "Temperature"="Temperature", "Camera Handle"=w113) -> ("error out"=w103:errorcluster, "String"=w110:string, "INI Flag"=w109:bool, "Camera Handle"=w98:u32)  [unwired: 5 in]
      n16 = local write "INI Flag"(w109) -> ()
      n17 = local write "Error Codes"(w110) -> ()
      n18 = call "ADC.vi"("ADC offset"="Offset", "ADC Gain"="Gain", "error in (no error)"=w103, "ADC Speed"="Speed", "Read Out port"="Readout Port", "Camera Handle"=w98) -> ("error out"=w96:errorcluster, "string"=w99:string, "INI Flag"=w100:bool, "Camera Handle"=w97:u32)  [unwired: 2 in]
      n19 = local write "INI Flag"(w100) -> ()
      n20 = local write "Error Codes"(w99) -> ()
      n21 = call "SHUTTER_CCD.vi"("Shutter State"="Shutter State", "error out"=w96, "Shutter Comp Time: Pre Open"="Close", "Shutter Comp Time: Post Open"="Open", "Camera Handle"=w97) -> ("error out"=w91:errorcluster, "String"=w90:string, "INI Flag"=w89:bool, "Camera Handle"=w92:u32)  [unwired: 3 in]
      n22 = local write "Error Codes"(w90) -> ()
      n23 = local write "INI Flag"(w89) -> ()
      n24 = Not(x="Skip Serial Register Clean") -> (.not. x?=w8:bool)
      n25 = call "CLEAN.vi"("Number of Strips Per Clear"="Number of Strips per Clean", "Number of Clears"="Number of Clean/Clears cycles", "Number of Minimum blocks"="Number of Minimum Blocks", "Minimum Block Size"="Minium Block Size", "error out"=w91, "Continous Clean"="Continous Cleans", "Skip Serial Reg Clean"=w8, "Camera Handle"=w92) -> ("error out 2"=w80:errorcluster, "String"=w83:string, "INI Flag"=w82:bool, "CameraHandle"=w81:u32)
      n26 = call "CUSTOM_CHIP.vi"("Camera Handle"=w81, "Window Size"="Kinetics Window Height", "TriggerMode"=w70, "Vertical Clock"="Vertical Timing Index", "error out"=w80, "Pre Y"="Pre Y", "Pre X"="Pre X", "Enable / Disable Custom Chip"=w6, "ReadOut Mode"=w71, "Post Y"="Post Y", "Post X"="Post X", "Parallel (Y) Size"="Active Y Size", "Serial (X) Size"="Active X Size") -> ("Camera Handle"=w67:u32, "INI Flag"=w73:bool, "String"=w72:string, "error out"=w66:errorcluster)  [unwired: 3 in]
      n27 = local write "INI Flag"(w73) -> ()
      n28 = local write "Error Codes"(w72) -> ()
      n29 = call "LOGIC.vi"("error out"=w66, "Invert"="Invert", "Logic Output"="Logic Output", "Camera Handle"=w67) -> ("error out 2"=w60:errorcluster, "String"=w62:string, "INI Flag"=w63:bool, "Camera Handle"=w59:u32)  [unwired: 4 in]
      n30 = local write "INI Flag"(w63) -> ()
      n31 = local write "Error Codes"(w62) -> ()
      n32 = case shown="True" w61 {
        tunnel: [w198 w214] -> w50
        tunnel: [w197 w213] -> w51
        tunnel: w60 -> [w195 w211]
        tunnel: [w196 w210] -> w58
        frame False {
          n33 = global read "CamHandle.vi" "X dimension"() -> (w199:u32)
          n34 = property on="Readut Mode" class="Ring (strict)"(error in=w195) -> (error out=w194:errorcluster, "Value"=w200:u16)  [unwired: 1 in, 1 out]
          n35 = Equal?(x=w200, y=10) -> (x = y?=w201:bool)
          n36 = case shown="True" w201 {
            tunnel: w199 -> [w205 w209]
            tunnel: [w205 w209] -> w198
            tunnel: [w204 w208] -> w197
            tunnel: [w203 w207] -> w196
            tunnel: w194 -> [w203 w206]
            frame False {
              n37 = global read "CamHandle.vi" "Y dimension"() -> (w204:u32)
            }
            frame True {
              n38 = property on="Kinetics Window Height" class="DigNum (strict)"(error in=w206) -> (error out=w207:errorcluster, "Value"=w208:u32)  [unwired: 1 in, 1 out]
            }
          }
        }
        frame True {
          n39 = property on="Active X Size" class="DigNum (strict)"(error in=w211) -> (error out=w212:errorcluster, "Value"=w214:u32)  [unwired: 1 in, 1 out]
          n40 = property on="Active Y Size" class="DigNum (strict)"(error in=w212) -> (error out=w210:errorcluster, "Value"=w213:u32)  [unwired: 1 in, 1 out]
        }
      }
      "X Size ROI" <- w50
      "Y Size ROI" <- w51
      n41 = call "ROI.vi"("Camera Handle"=w59, "Y Start"="Y Start", "Y End"="Y End", "Y Bin"="Y Bin", "error in"=w58, "X Start"="X Start", "X End"="X End", "X Bin"="X Bin") -> ("Camera Handle"=w15:u32, "INI Flag"=w49:bool, "String"=w2:string, "error out"=w14:errorcluster)  [unwired: 4 in]
      n42 = local write "Error Codes"(w2) -> ()
      n43 = local write "INI Flag"(w49) -> ()
      n44 = local write "INI Flag"(w82) -> ()
      n45 = local write "Error Codes"(w83) -> ()
      n46 = property class="TabCtl (strict)"("DisabledEnum"=T2."Disabled and Grayed Out" ("Disabled")) -> ()  [unwired: 2 in, 2 out]
      n47 = case shown="True" "INI Flag" {
        tunnel: w14 -> [w137 w165]
        tunnel: [w137 w163] -> w16
        tunnel: w15 -> [w135 w139]
        tunnel: [w135 w138] -> w13
        frame False {
          n48 = Wait Until Next ms Multiple(millisecond multiple=u32 10) -> ()  [unwired: 1 out]
        }
        frame True {
          n49 = call <userlib>:"CameraInitialize.vi"("error in"=w165, "Camera Handle"=w139) -> ("error out"=w166:errorcluster, "Camera Handle"=w138:u32)
          n50 = property on="Shutter State" class="Ring (strict)"() -> ("Value"=w187:u16)  [unwired: 2 in, 2 out]
          n51 = property on="Open" class="DigNum (strict)"() -> ("Value"=w188:u32)  [unwired: 2 in, 2 out]
          n52 = property on="Close" class="DigNum (strict)"() -> ("Value"=w189:u32)  [unwired: 2 in, 2 out]
          n53 = property on="Logic Output" class="Ring (strict)"() -> ("Value"=w190:u16)  [unwired: 2 in, 2 out]
          n54 = property on="Invert" class="Bool (strict)"() -> ("Value"=w191:bool)  [unwired: 2 in, 2 out]
          n55 = property on="Pre Y" class="DigNum (strict)"() -> ("Value"=w160:u32)  [unwired: 2 in, 2 out]
          n56 = property on="Post Y" class="DigNum (strict)"() -> ("Value"=w152:u32)  [unwired: 2 in, 2 out]
          n57 = property on="Active Y Size" class="DigNum (strict)"() -> ("Value"=w155:u32)  [unwired: 2 in, 2 out]
          n58 = property on="Pre X" class="DigNum (strict)"() -> ("Value"=w159:u32)  [unwired: 2 in, 2 out]
          n59 = property on="Post X" class="DigNum (strict)"() -> ("Value"=w153:u32)  [unwired: 2 in, 2 out]
          n60 = property on="Active X Size" class="DigNum (strict)"() -> ("Value"=w158:u32)  [unwired: 2 in, 2 out]
          n61 = property on="Enable  Custom Chip" class="Bool (strict)"() -> ("Value"=w157:bool)  [unwired: 2 in, 2 out]
          n62 = property on="Vertical Timing Index" class="DigNum (strict)"() -> ("Value"=w156:u32)  [unwired: 2 in, 2 out]
          n63 = Bundle By Name(cluster=T7 {"Shutter State"=2, "Open Comp Time "=0, "Close Comp Time"=0, "Logic Out Setting"=1, "Logic Out Invert"=FALSE} ("Shutter and Logic Out"), "Shutter State"=w187, "Open Comp Time"=w188, "Close Comp Time"=w189, "Logic Out Setting"=w190, "Logic Out Invert"=w191) -> (w192:T7)
          n64 = property on="Speed" class="DigNum (strict)"() -> ("Value"=w184:i32)  [unwired: 2 in, 2 out]
          n65 = property on="Gain" class="Ring (strict)"() -> ("Value"=w183:i32)  [unwired: 2 in, 2 out]
          n66 = property on="Offset" class="DigNum (strict)"() -> ("Value"=w181:i32)  [unwired: 2 in, 2 out]
          n67 = property on="Readout Port" class="Ring (strict)"() -> ("Value"=w179:i32)  [unwired: 2 in, 2 out]
          n68 = property on="Number of Clean/Clears cycles" class="DigNum (strict)"() -> ("Value"=w178:u32)  [unwired: 2 in, 2 out]
          n69 = property on="Number of Strips per Clean" class="DigNum (strict)"() -> ("Value"=w177:u32)  [unwired: 2 in, 2 out]
          n70 = property on="Minium Block Size" class="DigNum (strict)"() -> ("Value"=w175:u32)  [unwired: 2 in, 2 out]
          n71 = property on="Number of Minimum Blocks" class="DigNum (strict)"() -> ("Value"=w176:u32)  [unwired: 2 in, 2 out]
          n72 = property on="Continous Cleans" class="Bool (strict)"() -> ("Value"=w180:bool)  [unwired: 2 in, 2 out]
          n73 = property on="Skip Serial Register Clean" class="Bool (strict)"() -> ("Value"=w182:bool)  [unwired: 2 in, 2 out]
          n74 = Bundle By Name(cluster=T4 {"Pre Y"=0, "Post Y"=0, "Active Y"=0, "Pre X"=0, "Post X"=0, "Active X"=0, "Custom Chip Enabled"=FALSE, "Vertical Timing Index"=0} ("Custom Chip"), "Pre Y"=w160, "Post Y"=w152, "Active Y"=w155, "Pre X"=w159, "Post X"=w153, "Active X"=w158, "Custom Chip Enabled"=w157, "Vertical Timing Index"=w156) -> (w154:T4)
          n75 = Bundle By Name(cluster=T6 {"ADC Speed"=-2, "ADC Gain"=-1, "ADC Offset"=-1, "Readout Port"=-1, "Num Cleans"=1, "Num Strips per Clean"=10, "Mini Block Size"=2, "Num Min Blocks"=3, "Continous Cleans"=FALSE, "Skip Serial Reg Clean"=FALSE} ("ADC and Cleans"), "ADC Speed"=w184, "ADC Gain"=w183, "ADC Offset"=w181, "Readout Port"=w179, "Num Cleans"=w178, "Num Strips per Clean"=w177, "Mini Block Size"=w175, "Num Min Blocks"=w176, "Continous Cleans"=w180, "Skip Serial Reg Clean"=w182) -> (w185:T6)
          n76 = property on="Camera Number" class="DigNum (strict)"() -> ("Value"=w167:u32)  [unwired: 2 in, 2 out]
          n77 = property on="Camera Number" class="DigNum (strict)"() -> ("Value"=w149:u32)  [unwired: 2 in, 2 out]
          n78 = property on="X Start" class="DigNum (strict)"() -> ("Value"=w147:u32)  [unwired: 2 in, 2 out]
          n79 = property on="X End" class="DigNum (strict)"() -> ("Value"=w146:u32)  [unwired: 2 in, 2 out]
          n80 = property on="X Bin" class="DigNum (strict)"() -> ("Value"=w145:u32)  [unwired: 2 in, 2 out]
          n81 = property on="Y Start" class="DigNum (strict)"() -> ("Value"=w144:u32)  [unwired: 2 in, 2 out]
          n82 = property on="Y End" class="DigNum (strict)"() -> ("Value"=w143:u32)  [unwired: 2 in, 2 out]
          n83 = property on="Y Bin" class="DigNum (strict)"() -> ("Value"=w142:u32)  [unwired: 2 in, 2 out]
          n84 = property on="Exposure" class="DigNum (strict)"() -> ("Value"=w168:dbl)  [unwired: 2 in, 2 out]
          n85 = property on="Collection Mode" class="Ring (strict)"() -> ("Value"=w169:u32)  [unwired: 2 in, 2 out]
          n86 = property on="Timing Mode" class="Ring (strict)"() -> ("Value"=w170:u32)  [unwired: 2 in, 2 out]
          n87 = property on="Trigger Edge" class="Ring (strict)"() -> ("Value"=w171:u32)  [unwired: 2 in, 2 out]
          n88 = property on="Temperature" class="DigNum (strict)"() -> ("Value"=w172:dbl)  [unwired: 2 in, 2 out]
          n89 = Bundle By Name(cluster=T3 {"Camera Number"=0, "ROI Number"=0, "X Start"=0, "X End"=0, "X Bin"=0, "Y Start"=0, "Y End"=0, "Y Bin"=0} ("ROI Values"), "Camera Number"=w149, "ROI Number"=1, "X Start"=w147, "X End"=w146, "X Bin"=w145, "Y Start"=w144, "Y End"=w143, "Y Bin"=w142) -> (w141:T3)
          n90 = Bundle By Name(cluster=T5 {"Exposure"=0.001, "Collection Mode"=1, "Timing Mode"=1, "Trigger Edge"=1, "Temperature"=-10.0} ("Timing and Temperature"), "Exposure"=w168, "Collection Mode"=w169, "Timing Mode"=w170, "Trigger Edge"=w171, "Temperature"=w172) -> (w173:T5)
          n91 = call "CCD_cinfig_to_INP.vi"("Timing and Temperature"=w173, "Custom Chip"=w154, "ADC and Cleans"=w185, "error in (no error)"=w166, "Shutter and Logic Out"=w192, "Camera Number"=w167) -> ("error out"=w164:errorcluster)  [unwired: 5 in]
          n92 = call "ROI_to_INP.vi"("error in (no error)"=w164, "Show Message"=FALSE, "ROI Values"=w141) -> ("error out"=w151:errorcluster)  [unwired: 8 in]
          n93 = property on="INI Flag" class="Bool (strict)"(error in=w151, "Value"=FALSE) -> (error out=w163:errorcluster)  [unwired: 1 in, 1 out]
        }
      }
      n94 = call <userlib>:"CameraExperiment.vi"("Number of Accumulations"=1, "Acquire / Focus Flag"=w17, "error in"=w16, "Number of Images"=w19, "Exposure (sec)"=w22, "Camera Handle"=w13) -> ("error out"=w24:errorcluster, "Camera Handle"=w23:u32)
      n95 = call <userlib>:"CameraInitialize.vi"("error in"=w24, "Camera Handle"=w23) -> ("error out"=w26:errorcluster, "Camera Handle"=w25:u32)
      n96 = call <userlib>:"CameraADCget.vi"("Camera handle"=w25, "error in (no error)"=w26) -> ("Bit Depth"=→"Bit Depth":i32, "Pixel Time"=→"Pixel Time":i32, "Readout Port"=→"ReadOut Port":i32, "ADC Offset"=→"ADC Offset":i32, "Camera handle"=w41:u32, "ADC Speed"=→"ADC Speed":i32, "ADC Gain"=→"ADC Gain":i32, "error out"=w42:errorcluster)
      n97 = while {
        shift-right: [w132] -> w39
        shift-left: w42 -> [w134]
        shift-right: [w131] -> w38
        shift-left: w41 -> [w133]
        stop <- w127 stop-if-true
        n98 = local read "Temperature"() -> (w129:dbl)
        n99 = Wait (ms)(milliseconds to wait=u32 1000) -> ()  [unwired: 1 out]
        n100 = call <userlib>:"CameraGetTemp.vi"("Camera Handle"=w133, "error in (no error)"=w134) -> ("Camera Handle"=w131:u32, "Temperature"=w130:dbl, "error out"=w132:errorcluster)
        "Temperature" <- w130
        n101 = Less Or Equal?(x=w130, y=w129) -> (x <= y?=w125:bool)
        n102 = Or(x="Bypass Cooling", y=w125) -> (x .or. y?=w127:bool)
      }
      n103 = call <userlib>:"CameraGetVar.vi"("error in"=w39, "Parameter ID"=w40, "Camera Handle"=w38) -> ("error out"=w32:errorcluster, "Value"=→"Readout Time":dbl, "Camera Handle"=w30:u32)
      n104 = call <userlib>:"CameraGetVar.vi"("error in"=w32, "Parameter ID"=252, "Camera Handle"=w30) -> ("error out"=w31:errorcluster, "Value"=→"Frame Rate":dbl, "Camera Handle"=w29:u32)
      n105 = call <userlib>:"CameraGetCustomChip.vi"("Camera Handle"=w29, "error in (no error)"=w31) -> ("Camera Handle"=w36:u32, "Custum chip Enable/Disable status"=w4:bool, "error out"=w35:errorcluster)  [unwired: 1 out]
      n106 = Not(x=w4) -> (.not. x?=→"Custom Chip Enabled":bool)
      n107 = call <userlib>:"CameraGetVertClkInfo.vi"("Camera Handle"=w36, "error in (no error)"=w35) -> ("Camera Handle"=→"Camera Handle":u32, "VertClk index"=→"Vertical Index":u32, "Real Clock Value"=→"Vertical Timing":dbl, "error out"=w21:errorcluster)  [unwired: 2 out]
      n108 = call "Error_Filter.vi"("error in (no error)"=w21, "Error Numbers To Filter"="5011") -> ("error out"=→"error out":errorcluster)  [unwired: 9 in]
    }
    frame #1 {
      n109 = while {
        stop <- w218 stop-if-true
        n110 = local read "Camera Handle"() -> (w219:u32)
        n111 = local read "error out"() -> (w220:errorcluster)
        n112 = stacked-sequence {
          seq-local: [_ w330 _ _] -> [_ _ w429 _]
          seq-local: [_ w329 _ _] -> [_ _ w431 _]
          seq-local: [w231 _ _ _] -> [_ w327 _ _]
          seq-local: [w232 _ _ _] -> [_ w328 _ _]
          tunnel: w219 -> [w229 _ _ w616]
          tunnel: w220 -> [w235 _ _ w617]
          tunnel: "?" -> [w233 w335 w435 w619]
          tunnel: "Number of Images" -> [_ w333 w432 w615]
          tunnel: "Timepoints" -> [_ _ w425 _]
          tunnel: [_ _ w428 _] -> _
          tunnel: [_ _ w427 _] -> _
          tunnel: "# of Sets" -> [_ _ w426 _]
          tunnel: [_ _ w422 _] -> w216
          frame #0 {
            n113 = Equal?(x=w233, y=enum32{"RUN", "FOCUS", "FSRS", "SPECTROGRAPH"}."RUN") -> (x = y?=w230:bool)
            n114 = case shown="False" "?" {
              tunnel: w235 -> [w241 w274]
              tunnel: [w238 w277] -> w231
              tunnel: [w240 w276] -> w232
              tunnel: w230 -> [_ _]
              tunnel: w229 -> [w239 w275]
              tunnel: "Exposure Time (s)" -> [w237 w272]
              frame False {
                n115 = case shown="True" "?" {
                  tunnel: w241 -> [w243 w255]
                  tunnel: [w243 w254] -> w240
                  tunnel: w239 -> [w242 w256]
                  tunnel: [w242 w253] -> w238
                  tunnel: w237 -> [_ w257]
                  frame False {
                  }
                  frame True {
                    n116 = Path To String(path="file path") -> (string=w249:string)
                    n117 = Concatenate Strings(w249, "\\" ("string"), "File_name", "_" ("string")) -> (w244:string)
                    n118 = for {
                      N: "# of Frames" -> [_]
                      tunnel: w257 -> [w271]
                      tunnel: w256 -> [w270]
                      tunnel: w255 -> [w269]
                      tunnel: [w268] -> w254
                      tunnel: [w267] -> w253
                      tunnel: "# of spectrum per frame" -> [w266]
                      tunnel: w244 -> [w263]
                      i -> [w260]
                      n119 = Number To Decimal String(number=w260) -> (decimal integer string=w262:string)  [unwired: 1 in]
                      n120 = call "avarage_images.vi"("error in (no error)"=w269, "Exposure Time (s)"=w271, "Number of Images"=w266, "Camera Handle"=w270) -> ("error out"=w268:errorcluster, "Camera Handle"=w267:u32, "Waveform Graph"=w259:i32[])  [unwired: 3 in, 2 out]
                      n121 = Concatenate Strings(w263, w262) -> (w261:string)
                      n122 = Reverse 1D Array(array=w259) -> (reversed array=w258:i32[])
                      n123 = String To Path(string=w261) -> (path=w264:path)
                      n124 = local write item#16(w258) -> ()
                      n125 = call-poly <vilib>:"Write To Spreadsheet File.vi"("transpose? (no:F)"=TRUE, "1D data"=w258, "file path (dialog if empty)"=w264) -> ()  [unwired: 5 in, 1 out]
                    }
                    n126 = local write "Ready to Run"(FALSE ("PyLoN Ready")) -> ()
                  }
                }
              }
              frame True {
                w279 = u32 1  # acquire focus mode
                w280 = u32 1  # Software accumulation
                # "focus mode (1) ->"
                # "This is similar to \"Run\"  in Lightfield\nTrigger mode= internal"
                n127 = call "ExSubImageCreate.vi"("Camera Handle"=w275, "error in (no error)"=w274) -> ("Camera Handle"=w281:u32, "Data Handle"=w287:u32, "error out"=w282:errorcluster)
                n128 = Bundle("acquire focus mode"=w279, "Exposure Time (s)"=w272, 1, "Software accumulation"=w280) -> (w278:T8)  [unwired: 1 in]
                n129 = call "ExSubInitCam.vi"("error in (no error)"=w282, "Camera Information"=w278, "Camera Handle"=w281) -> ("error out"=w283:errorcluster, "Camera Handle"=w284:u32)
                n130 = call <userlib>:"CameraStart.vi"("error in"=w283, "Camera Handle"=w284) -> ("error out"=w285:errorcluster, "Camera Handle"=w286:u32)
                n131 = local write "Ready to Run"(FALSE ("PyLoN Ready")) -> ()
                n132 = while {
                  tunnel: [w302] -> w288
                  tunnel: [w301] -> w290
                  tunnel: [w300] -> w289
                  tunnel: w285 -> [w299]
                  tunnel: w286 -> [w298]
                  tunnel: w287 -> [w297]
                  stop <- "?" stop-if-true
                  n133 = call <userlib>:"CameraCheckData.vi"("Camera Handle"=w298, "error in"=w299) -> ("Camera Handle"=w304:u32, "Number Of Frames Available"=w306:i32, "error out"=w303:errorcluster)
                  n134 = Greater Than 0?(x=w306) -> (x > 0?=w305:bool)
                  n135 = case shown="True" w305 {
                    selector: w305 -> [w309 w323]
                    tunnel: w304 -> [w307 w325]
                    tunnel: w303 -> [w310 w324]
                    tunnel: [w309 w323] -> _
                    tunnel: [w310 w322] -> w301
                    tunnel: w297 -> [w308 w316]
                    tunnel: [w308 w320] -> w302
                    tunnel: [w307 w319] -> w300
                    frame False {
                    }
                    frame True {
                      w321 = 1
                      n136 = call <userlib>:"CameraGetData.vi"("error in"=w324, "Image/Data Handle"=w316, "Camera Handle"=w325) -> ("error out"=w318:errorcluster, "Image/Data Handle"=w317:u32, "Camera Handle"=w319:u32)
                      n137 = call <userlib>:"ImageGetLineU16.vi"("Data Handle"=w317, "Y Position"=w321, "Z Position"=w321, "error in"=w318) -> ("Array u16"=w315:u16[], "Data Handle"=w320:u32, "error out"=w322:errorcluster)
                      n138 = Delete From Array(array=w315, length=2, index=0) -> (array with subset deleted=w312:u16[])  [unwired: 1 out]
                      n139 = Reverse 1D Array(array=w312) -> (reversed array=→"?":u16[])
                    }
                  }
                }
                n140 = call <userlib>:"ImageDestroy.vi"("error in"=w290, "Data handle"=w288) -> ()  [unwired: 1 out]
                n141 = stacked-sequence {
                  tunnel: w290 -> [w295]
                  tunnel: w289 -> [w294]
                  tunnel: [w293] -> w276
                  tunnel: [w292] -> w277
                  frame #0 {
                    n142 = call <userlib>:"CameraStop.vi"("error in"=w295, "Camera Handle"=w294) -> ("error out"=w293:errorcluster, "Camera Handle"=w292:u32)
                    n143 = call <vilib>:"Beep.vi"() -> ()  [unwired: 12 in]
                  }
                }
              }
            }
            "Ready to Run" <- TRUE
          }
          frame #1 {
            n144 = Equal?(x=w335, y=enum32{"RUN", "FOCUS", "FSRS", "SPECTROGRAPH"}."FOCUS") -> (x = y?=w331:bool)
            n145 = And(x=w331, y="?") -> (x .and. y?=w334:bool)
            n146 = case shown="False" w334 {
              tunnel: w327 -> [w343 w394]
              tunnel: [w339 w393] -> w330
              tunnel: w328 -> [w341 w392]
              tunnel: w333 -> [w342 w391]
              tunnel: [w340 w390] -> w329
              tunnel: w331 -> [w336 _]
              frame False {
                n147 = And(x=w336, y="?") -> (x .and. y?=w338:bool)
                n148 = case shown="False" w338 {
                  tunnel: w343 -> [w346 w373]
                  tunnel: w342 -> [w347 w372]
                  tunnel: w341 -> [w348 w371]
                  tunnel: [w344 w370] -> w340
                  tunnel: [w345 w369] -> w339
                  tunnel: w336 -> [w349 _]
                  frame False {
                    n149 = And(x=w349, y="?") -> (x .and. y?=w351:bool)
                    n150 = case shown="True" w351 {
                      tunnel: w348 -> [w352 w358]
                      tunnel: w347 -> [_ w361]
                      tunnel: w346 -> [w353 w360]
                      tunnel: [w353 w356] -> w345
                      tunnel: [w352 w357] -> w344
                      frame False {
                      }
                      frame True {
                        # "Acquire"
                        n151 = Initialize Array(0.0, u32 1340) -> (w359:dbl[])
                        n152 = local read "FLIP SPECTRA"() -> (w363:bool)
                        n153 = call "PyLoN_data.vi"("Number of Images"=w361, "error in (no error)"=w358, "PumpOffBkgd"=w359, "PumpOnBkgd"=w359, "Camera Handle"=w360) -> ("error out"=w357:errorcluster, "Camera Handle 2"=w356:u32, "Raman_Gain"=w355:dbl[])  [unwired: 1 in, 3 out]
                        n154 = local write "Ready to Run"(FALSE ("Ready to Run")) -> ()
                        n155 = case shown="False" w363 {
                          tunnel: w355 -> [w366 w368]
                          tunnel: [w366 w367] -> w362
                          frame False {
                          }
                          frame True {
                            n156 = Reciprocal(x=w368) -> (1/x=w367:dbl[])
                          }
                        }
                        n157 = local write "Spectra"(w362) -> ()
                      }
                    }
                  }
                  frame True {
                    # "Winspec"
                    n158 = while {
                      tunnel: w373 -> [w380]
                      tunnel: w372 -> [w381]
                      tunnel: [w375] -> w369
                      tunnel: w371 -> [w379]
                      tunnel: [w378] -> w370
                      stop <- w384 stop-if-true
                      n159 = local read item#11() -> (w384:bool)
                      n160 = Initialize Array(0.0, u32 1340) -> (w376:dbl[])
                      n161 = local read "FLIP SPECTRA"() -> (w383:bool)
                      n162 = call "PyLoN_data.vi"("Number of Images"=w381, "error in (no error)"=w379, "PumpOffBkgd"=w376, "PumpOnBkgd"=w376, "Camera Handle"=w380) -> ("error out"=w378:errorcluster, "Pump_Off"=w377:dbl[], "Camera Handle 2"=w375:u32)  [unwired: 1 in, 3 out]
                      n163 = local write "Ready to Run"(FALSE ("Ready to Run")) -> ()
                      n164 = case shown="False" w383 {
                        tunnel: w377 -> [w387 w388]
                        tunnel: [w387 w389] -> w382
                        frame False {
                        }
                        frame True {
                          n165 = Reciprocal(x=w388) -> (1/x=w389:dbl[])
                        }
                      }
                      n166 = local write "Spectra"(w382) -> ()
                    }
                  }
                }
              }
              frame True {
                # "Focus"
                n167 = while {
                  tunnel: w392 -> [w411]
                  tunnel: w391 -> [w412]
                  tunnel: [w410] -> w390
                  tunnel: w394 -> [w413]
                  tunnel: [w408] -> w393
                  stop <- "?" stop-if-true
                  n168 = property on="Spectra" class="WFGraph (strict)"("Active Cursor"=u32 1) -> (error out=w403:errorcluster)  [unwired: 2 in, 1 out]
                  n169 = property on="Spectra" class="WFGraph (strict)"("Active Cursor"=u32 0) -> (error out=w404:errorcluster)  [unwired: 2 in, 1 out]
                  n170 = Initialize Array(0.0, u32 1340) -> (w409:dbl[])
                  n171 = call "PyLoN_data.vi"("Number of Images"=w412, "error in (no error)"=w411, "PumpOffBkgd"=w409, "PumpOnBkgd"=w409, "Camera Handle"=w413) -> ("error out"=w410:errorcluster, "Pump_Off"=→"?":dbl[], "Camera Handle 2"=w408:u32, "Raman_Gain"=w407:dbl[])  [unwired: 1 in, 2 out]
                  n172 = property on="Spectra" class="WFGraph (strict)"(error in=w403) -> ("Cursor.Cursor Y"=w401:dbl)  [unwired: 1 in, 2 out]
                  n173 = property on="Spectra" class="WFGraph (strict)"(error in=w404) -> ("Cursor.Cursor Y"=w402:dbl)  [unwired: 1 in, 2 out]
                  n174 = local read "FLIP SPECTRA"() -> (w415:bool)
                  n175 = Subtract(x=w402, y=w401) -> (x-y=w400:dbl)
                  n176 = Absolute Value(x=w400) -> (abs(x)=w399:dbl)
                  n177 = local write "Ready to Run"(FALSE ("Ready to Run")) -> ()
                  n178 = Multiply(x=w399, y=100.0) -> (x*y=→"Gain":dbl)
                  n179 = case shown="False" w415 {
                    tunnel: w407 -> [w419 w421]
                    tunnel: [w419 w420] -> w414
                    frame False {
                    }
                    frame True {
                      n180 = Reciprocal(x=w421) -> (1/x=w420:dbl[])
                    }
                  }
                  "Spectra" <- w414
                }
              }
            }
          }
          frame #2 {
            n181 = Array Size(array=w425) -> (size(s)=w424:i32)
            n182 = Equal?(x=w435, y=enum32{"RUN", "FOCUS", "FSRS", "SPECTROGRAPH"}."FSRS") -> (x = y?=w433:bool)
            n183 = And(x="?", y=w433) -> (x .and. y?=w434:bool)
            n184 = case shown="True" w434 {
              tunnel: w432 -> [_ w447]
              tunnel: w429 -> [w437 w446]
              tunnel: w431 -> [w438 w442]
              tunnel: w425 -> [_ w445]
              tunnel: [w437 w444] -> w428
              tunnel: [w438 w443] -> w427
              tunnel: w426 -> [_ w441]
              tunnel: w424 -> [_ w440]
              tunnel: [FALSE w439] -> w422
              frame False {
              }
              frame True {
                n185 = for {
                  N: w441 -> [_]
                  tunnel: w447 -> [w455]
                  tunnel: w446 -> [w454]
                  tunnel: w445 -> [w453]
                  tunnel: [w452] -> w444
                  tunnel: [w451] -> w443
                  tunnel: w442 -> [w450]
                  tunnel: w440 -> [w449]
                  tunnel: [w448] -> w439
                  n186 = stacked-sequence {
                    seq-local: [w458 _] -> [_ w469]
                    tunnel: w455 -> [_ w468]
                    tunnel: w454 -> [_ w467]
                    tunnel: [_ w463] -> _
                    tunnel: w453 -> [w456 w466]
                    tunnel: [_ w465] -> w451
                    tunnel: [_ w464] -> w452
                    tunnel: w450 -> [_ w463]
                    tunnel: w449 -> [_ w462]
                    tunnel: [_ w461] -> w448
                    frame #0 {
                      n187 = Array Size(array=w456) -> (size(s)=w460:i32)
                      n188 = call "randomize.vi"("Input array"=w456) -> ("Output array"=w457:dbl[])
                      n189 = Quotient & Remainder(x=w460, y="#Ground per set") -> (floor(x/y)=w458:u32)  [unwired: 1 out]
                      n190 = local write "Timepoints"(w457) -> ()
                    }
                    frame #1 {
                      n191 = for {
                        N: w462 -> [_]
                        tunnel: w469 -> [w477]
                        tunnel: w468 -> [w476]
                        tunnel: w467 -> [w475]
                        tunnel: w466 -> [w474]
                        tunnel: [w473] -> w465
                        tunnel: [w472] -> w464
                        tunnel: w463 -> [w471]
                        tunnel: [w470] -> w461
                        i -> [w478]
                        n192 = stacked-sequence {
                          seq-local: [w480 _] -> [_ w544]
                          seq-local: [w481 _] -> [_ w545]
                          seq-local: [w479 _] -> [_ w543]
                          tunnel: w478 -> [w482 w546]
                          tunnel: w477 -> [w487 _]
                          tunnel: w476 -> [w485 w548]
                          tunnel: w475 -> [w484 _]
                          tunnel: w471 -> [w483 _]
                          tunnel: w474 -> [_ w547]
                          tunnel: [_ w542] -> w473
                          tunnel: [_ w541] -> w472
                          tunnel: [_ w540] -> w470
                          frame #0 {
                            n193 = Quotient & Remainder(x=w482, y=w487) -> (x-y*floor(x/y)=w488:u32, floor(x/y)=w486:u32)
                            n194 = Equal To 0?(x=w488) -> (x = 0?=w489:bool)
                            n195 = case shown="True" w489 {
                              tunnel: w486 -> [_ w501]
                              tunnel: w485 -> [_ w505]
                              tunnel: w484 -> [w491 w504]
                              tunnel: w483 -> [w490 w503]
                              tunnel: [w491 w494] -> w480
                              tunnel: [w490 w493] -> w481
                              tunnel: w482 -> [_ w502]
                              tunnel: [_ w492] -> w479
                              frame False {
                              }
                              frame True {
                                n196 = flat-sequence {
                                tunnel: w505 -> [w526]
                                tunnel: w504 -> [w525]
                                tunnel: w503 -> [w524]
                                tunnel: w502 -> [w513]
                                tunnel: w501 -> [w511]
                                tunnel: [w523] -> w500
                                tunnel: [w522] -> w499
                                tunnel: [w506] -> w498
                                tunnel: [w519] -> w497
                                tunnel: [w508] -> w496
                                tunnel: [w507] -> w495
                                tunnel: w500 -> [w532]
                                tunnel: w499 -> [w531]
                                tunnel: w498 -> [w535]
                                tunnel: w497 -> [w534]
                                tunnel: w496 -> [w536]
                                tunnel: w495 -> [w530]
                                tunnel: [w532] -> w494
                                tunnel: [w531] -> w493
                                tunnel: [w530] -> w492
                                frame #0 {
                                w512 = "_" ("string")
                                n197 = local read "FLIP SPECTRA"() -> (w521:bool)
                                n198 = call "PyLoN_data.vi"("Number of Images"=w526, "error in (no error)"=w524, "Camera Handle"=w525) -> ("error out"=w522:errorcluster, "Pump_Off"=w519:dbl[], "Pump_On"=w506:dbl[], "Camera Handle 2"=w523:u32, "Raman_Gain"=w507:dbl[])  [unwired: 3 in, 1 out]
                                "?" <- w506
                                n199 = Format Into String(w513) -> (resulting string=w514:string)  [unwired: 3 in, 1 out]
                                n200 = Format Into String(w511) -> (resulting string=w510:string)  [unwired: 3 in, 1 out]
                                n201 = case shown="False" w521 {
                                tunnel: w507 -> [w527 w529]
                                tunnel: [w527 w528] -> w520
                                frame False {
                                }
                                frame True {
                                n202 = Reciprocal(x=w529) -> (1/x=w528:dbl[])
                                }
                                }
                                "?" <- w520
                                n203 = Path To String(path="File Path") -> (string=w518:string)
                                n204 = Concatenate Strings(w518, "\\" ("string"), "File Name", w512, w514, w512, w510, "gr" ("string")) -> (w508:string)
                                }
                                frame #1 {
                                n205 = String To Path(string=w536) -> (path=w537:path)
                                n206 = Build Array(w530, w535, w534) -> (w533:dbl[][])
                                n207 = call-poly <vilib>:"Write To Spreadsheet File.vi"("transpose? (no:F)"=TRUE, "format (%.3f)"="%.7f", "2D data"=w533, "file path (dialog if empty)"=w537) -> ()  [unwired: 4 in, 1 out]
                                }
                                }
                              }
                            }
                          }
                          frame #1 {
                            n208 = stacked-sequence {
                              seq-local: [_ w567 _ _ _] -> [_ _ _ w588 _]
                              seq-local: [_ w570 _ _ _] -> [_ _ _ w587 w595]
                              seq-local: [_ w569 _ _ _] -> [_ _ _ w586 w593]
                              seq-local: [_ w568 _ _ _] -> [_ _ _ w585 _]
                              tunnel: w545 -> [_ w580 _ _ _]
                              tunnel: w544 -> [_ w579 _ _ _]
                              tunnel: w548 -> [_ w578 _ _ _]
                              tunnel: w547 -> [w558 w575 _ _ _]
                              tunnel: w546 -> [w557 w571 _ _ _]
                              tunnel: w543 -> [_ _ _ _ w596]
                              tunnel: [_ w566 _ _ _] -> w542
                              tunnel: [_ w565 _ _ _] -> w541
                              tunnel: [w549 _ _ _ _] -> w540
                              frame #0 {
                                n209 = Index Array(array=w558, index=w557) -> (element=w556:dbl)
                                n210 = Multiply(x=w556, y=0.00015) -> (x*y=w560:dbl)
                                n211 = Add(x=w560, y="t0 position") -> (x+y=w554:dbl)
                                n212 = Absolute Value(x=w554) -> (abs(x)=w551:dbl)
                                n213 = In Range and Coerce(upper limit=49.9, x=w551, lower limit=0.0) -> (In Range?=w550:bool)  [unwired: 1 out]
                                n214 = case shown="False" w550 {
                                tunnel: w554 -> [_ _]
                                tunnel: [w561 FALSE] -> w549
                                frame False {
                                n215 = One Button Dialog(message="Stage Out of Range", button name ("OK")="OK") -> (true=w561:bool)
                                }
                                frame True {
                                }
                                }
                              }
                              frame #1 {
                                n216 = Index Array(array=w575, index=w571) -> (element=w574:dbl)
                                n217 = call "tppathcr.vi"("input"=w574) -> ("out"=w573:string)
                                n218 = local read "File Path"() -> (w577:path)
                                n219 = local read "File Name"() -> (w576:string)
                                n220 = call "PyLoN_data.vi"("Number of Images"=w578, "error in (no error)"=w580, "Camera Handle"=w579) -> ("error out"=w566:errorcluster, "Pump_Off"=w568:dbl[], "Pump_On"=w569:dbl[], "Camera Handle 2"=w565:u32, "Raman_Gain"=w570:dbl[])  [unwired: 3 in, 1 out]
                                n221 = Format Into String(w571) -> (resulting string=w581:string)  [unwired: 3 in, 1 out]
                                n222 = Path To String(path=w577) -> (string=w584:string)
                                n223 = Concatenate Strings(w584, "\\" ("string"), w576, "_" ("string"), w573, "exe" ("string"), w581) -> (w567:string)
                              }
                              frame #2 {
                              }
                              frame #3 {
                                n224 = String To Path(string=w588) -> (path=w590:path)
                                n225 = Build Array(w587, w586, w585) -> (w589:dbl[][])
                                n226 = call-poly <vilib>:"Write To Spreadsheet File.vi"("transpose? (no:F)"=TRUE, "format (%.3f)"="%.7f", "2D data"=w589, "file path (dialog if empty)"=w590) -> ()  [unwired: 4 in, 1 out]
                              }
                              frame #4 {
                                n227 = case shown="False" "Ground State\nSubstract?" {
                                tunnel: w596 -> [_ w605]
                                tunnel: w595 -> [w599 w604]
                                frame False {
                                n228 = local read "FLIP SPECTRA"() -> (w598:bool)
                                n229 = case shown="True" w598 {
                                tunnel: [w600 w602] -> w597
                                tunnel: w599 -> [w600 w601]
                                frame False {
                                }
                                frame True {
                                n230 = Reciprocal(x=w601) -> (1/x=w602:dbl[])
                                }
                                }
                                n231 = local write item#?(w597) -> ()
                                }
                                frame True {
                                n232 = local read "FLIP SPECTRA"() -> (w606:bool)
                                n233 = case shown="False" w606 {
                                tunnel: [w609 w614] -> w608
                                tunnel: w605 -> [w610 w611]
                                tunnel: [w610 w613] -> w607
                                tunnel: w604 -> [w609 w612]
                                frame False {
                                }
                                frame True {
                                n234 = Reciprocal(x=w612) -> (1/x=w614:dbl[])
                                n235 = Reciprocal(x=w611) -> (1/x=w613:dbl[])
                                }
                                }
                                n236 = Subtract(x=w608, y=w607) -> (x-y=w603:dbl[])
                                n237 = local write item#?(w603) -> ()
                                }
                                }
                                n238 = local write item#111(w593) -> ()
                              }
                            }
                          }
                        }
                      }
                    }
                  }
                }
              }
            }
          }
          frame #3 {
            n239 = Equal?(x=w619, y=enum32{"RUN", "FOCUS", "FSRS", "SPECTROGRAPH"}."SPECTROGRAPH") -> (x = y?=w620:bool)
            n240 = case shown="True" w620 {
              tunnel: w617 -> [_ w634]
              tunnel: w616 -> [_ w633]
              tunnel: w615 -> [_ w632]
              frame False {
              }
              frame True {
                # "Spectrometer Index\nThis is the number of the spectrometer\nas set in the spectrometer .ini file"
                n241 = call <userlib>:"InitToolkit.vi"("error in"="Spectrograph error in") -> ("error out"=w625:errorcluster)
                n242 = call "ExSubSpecOpenMultTurret.vi"("Camera Handle"=1, "Grating number"="Grating Number", "Grating speed"="Grating Speed", "error in (no error)"=w625, "Turret Number"="Turret Number") -> ("Spectrometer Handle"=w622:u32, "error out"=w624:errorcluster)  [unwired: 1 out]
                n243 = call <userlib>:"SpectSetMirror.vi"("error in"=w624, "Position"="Position", "Mirror"="Mirror Number", "Spectrometer Handle"=w622) -> ("error out"=w623:errorcluster, "Spectrometer Handle"=w621:u32)
                n244 = call <userlib>:"SpectSetWavelength.vi"("error in"=w623, "Wavelength"="Start Wavelength", "Spectrometer Handle"=w621) -> ("error out"=w644:errorcluster, "Spectrumeter Handle"=w643:u32)
                n245 = call "ExSubWaitSpec.vi"("error in (no error)"=w644, "Spectrometer Handle"=w643) -> ("error out"=w638:errorcluster, "Spectrometer handle"=w642:u32)
                n246 = case shown="True" "?" {
                  tunnel: w642 -> [w651 w671]
                  tunnel: "End Wavelength" -> [_ w670]
                  tunnel: "Increment Wavelength" -> [_ w669]
                  tunnel: "Start Wavelength" -> [_ w668]
                  tunnel: [w649 w667] -> w631
                  tunnel: w638 -> [w652 w666]
                  tunnel: w634 -> [_ w665]
                  tunnel: w633 -> [_ w664]
                  tunnel: w632 -> [_ w663]
                  tunnel: [w650 w662] -> w629
                  tunnel: "Center Wavelength" -> [w647 _]
                  frame False {
                    n247 = case shown="True" "?" {
                      tunnel: w652 -> [w654 w659]
                      tunnel: w651 -> [w653 w658]
                      tunnel: [w654 w657] -> w650
                      tunnel: [w653 w656] -> w649
                      tunnel: w647 -> [_ w655]
                      frame False {
                      }
                      frame True {
                        n248 = call <userlib>:"SpectSetWavelength.vi"("error in"=w659, "Wavelength"=w655, "Spectrometer Handle"=w658) -> ("error out"=w660:errorcluster, "Spectrumeter Handle"=w661:u32)
                        n249 = call "ExSubWaitSpec.vi"("error in (no error)"=w660, "Spectrometer Handle"=w661) -> ("error out"=w657:errorcluster, "Spectrometer handle"=w656:u32)
                      }
                    }
                  }
                  frame True {
                    n250 = while {
                      tunnel: w671 -> [w680]
                      tunnel: w669 -> [w683]
                      tunnel: w670 -> [w679]
                      shift-right: [w677] -> _
                      shift-left: w668 -> [w684]
                      tunnel: [w682] -> w667
                      tunnel: w666 -> [w681]
                      tunnel: w665 -> [w675]
                      tunnel: w664 -> [w674]
                      tunnel: w663 -> [w673]
                      tunnel: [w672] -> w662
                      stop <- w678 stop-if-true
                      n251 = Add(x=w684, y=w683) -> (x+y=w676:dbl)
                      n252 = stacked-sequence {
                        seq-local: [_ w698 _] -> [_ _ w715]
                        seq-local: [w686 _ _] -> [_ w697 _]
                        tunnel: [w693 _ _] -> w682
                        tunnel: w681 -> [w692 _ _]
                        tunnel: w680 -> [w690 _ _]
                        tunnel: w679 -> [w689 _ _]
                        tunnel: [w688 _ _] -> w677
                        tunnel: w676 -> [w687 _ _]
                        tunnel: w675 -> [_ w701 _]
                        tunnel: w674 -> [_ w700 _]
                        tunnel: w673 -> [_ w699 _]
                        tunnel: [_ w696 _] -> w672
                        frame #0 {
                          n253 = Max & Min(x=w687, y=w689) -> (min(x,y)=w688:dbl)  [unwired: 1 out]
                          n254 = call <userlib>:"SpectSetWavelength.vi"("error in"=w692, "Wavelength"=w688, "Spectrometer Handle"=w690) -> ("error out"=w691:errorcluster, "Spectrumeter Handle"=w694:u32)
                          n255 = Number To Fractional String(number=w688) -> (F-format string=→"Current Wavelength":string)  [unwired: 3 in]
                          n256 = call "ExSubWaitSpec.vi"("error in (no error)"=w691, "Spectrometer Handle"=w694) -> ("error out"=w686:errorcluster, "Spectrometer handle"=w693:u32)
                        }
                        frame #1 {
                          n257 = case shown="No Error" w697 {
                            selector: w697 -> [w705 w713]
                            tunnel: w701 -> [w710 _]
                            tunnel: w700 -> [w709 _]
                            tunnel: w699 -> [w708 _]
                            tunnel: [w706 _] -> w698
                            tunnel: [w705 w713] -> w696
                            frame No Error {
                              n258 = call "PyLoN_data.vi"("Number of Images"=w708, "error in (no error)"=w710, "Camera Handle"=w709) -> ("Pump_Off"=w707:dbl[], "Pump_On"=w703:dbl[], "Raman_Gain"=w702:dbl[])  [unwired: 3 in, 3 out]
                              n259 = case shown="\"FOCUS\", Default" "?" {
                                tunnel: w703 -> [_ w712]
                                tunnel: w702 -> [w711 _]
                                frame "FOCUS", Default {
                                n260 = local write item#105(w711) -> ()
                                }
                                frame "WINSPEC" {
                                "?" <- w712
                                }
                              }
                              n261 = Build Array(w703, w707, w702) -> (w706:dbl[][])
                            }
                            frame Error {
                            }
                          }
                        }
                        frame #2 {
                          n262 = case shown="True" "Save to a File" {
                            tunnel: w715 -> [_ w717]
                            frame False {
                            }
                            frame True {
                              n263 = local read "Current Wavelength"() -> (w720:string)
                              n264 = Path To String(path="File Path") -> (string=w725:string)
                              n265 = Concatenate Strings(w725, "\\" ("string"), "File Name", "_" ("string"), w720) -> (w719:string)
                              n266 = String To Path(string=w719) -> (path=w718:path)
                              n267 = call-poly <vilib>:"Write To Spreadsheet File.vi"("format (%.3f)"="%.7f", "2D data"=w717, "file path (dialog if empty)"=w718) -> ()  [unwired: 5 in, 1 out]
                            }
                          }
                        }
                      }
                      n268 = Greater?(x=w676, y=w679) -> (0:w678:bool)
                      n269 = Wait Until Next ms Multiple(millisecond multiple=50) -> ()  [unwired: 1 out]
                    }
                  }
                }
                "Spectrograph \nerror out" <- w629
                "Spectrometer\nhandle" <- w631
              }
            }
          }
        }
        n270 = Or(x=w220, y="?") -> (x .or. y?=w217:bool)
        n271 = Or(x=w217, y=w216) -> (x .or. y?=w218:bool)
      }
      n272 = property class="TabCtl (strict)"("DisabledEnum"=T2."Enabled" ("Disabled")) -> ()  [unwired: 2 in, 2 out]
    }
    frame #2 {
      n273 = local read "error out"() -> (w731:errorcluster)
      n274 = local read "Camera Handle"() -> (w730:u32)
      n275 = local read "Spectrometer\nhandle"() -> (w727:u32)
      n276 = local read "Spectrograph \nerror out"() -> (w728:errorcluster)
      n277 = local write "Ready to Run"(FALSE ("PyLoN Ready")) -> ()
      n278 = call <userlib>:"SpectClose.vi"("error in"=w728, "Spectrometer Handle"=w727) -> ("error out"=w729:errorcluster)
      n279 = call "ExSubCloseCamUnInit.vi"("error in (no error)"=w731, "Camera Handle"=w730) -> ("error out"=w733:errorcluster)
      n280 = local write "error out"(w733) -> ()
      n281 = call <userlib>:"UninitToolkit.vi"("error in"=w729) -> ("error out"=w726:errorcluster)
      n282 = local write "Spectrograph \nerror out"(w726) -> ()
    }
  }
